vi "Autopatch-v2.3_focus.vi"() -> ()   [LabVIEW 2018]
uses:
  <vilib>/userdefined/High Color/IMAQdx.ctl
  <vilib>/DAQmx/write.llb/DAQmx Write (Analog DBL 1Chan 1Samp).vi
  <vilib>/DAQmx/write.llb/DAQmx Write (Analog Wfm 1Chan NSamp).vi
  <vilib>/DAQmx/read.llb/DAQmx Read (Analog Wfm 1Chan NSamp).vi
  <vilib>/Analysis/baseanly.llb/Mean (DBL).vi
  <vilib>/DAQmx/create/channels.llb/DAQmx Create Channel (AO-Voltage-Basic).vi
  <vilib>/DAQmx/miscellaneous.llb/DAQmx Fill In Error Info.vi
  <vilib>/DAQmx/create/channels.llb/DAQmx Create Channel (AI-Voltage-Basic).vi
  <vilib>/DAQmx/configure/timing.llb/DAQmx Timing (Sample Clock).vi
  <vilib>/DAQmx/configure/trigger.llb/DAQmx Start Trigger (Digital Edge).vi
  <vilib>/Waveform/WDTOps.llb/WDT Waveform Duration DBL.vi
  <vilib>/addons/control/pid/pid.llb/PID (DBL).vi
  <vilib>/vision/driver/NI_Vision_Acquisition_Software.lvlib
  <resource>/objmgr/daqmx.rc
  <vilib>/Analysis/NI_AALBase.lvlib
  <vilib>/measure/NI_MABase.lvlib
  <vilib>/vision/NI_Vision_Development_Module.lvlib
  <vilib>/addons/control/pid/NI_PID_pid.lvlib
  <vilib>/Analysis/NI_AALPro.lvlib
panel:
  out "裁剪数组":i32[](array[numeric])
  in  "模板分数":sgl=650.0
  out "自动接触状态":i32
  in  "没有细胞":bool=TRUE
  out "x+y":sgl
  in  "z输入":dbl=24364.6
  in  "y输入":dbl=3592.0
  in  "x输入":dbl=-28569.0
  in  "二值化":bool=TRUE
  in  "背景图":path=path "D:/韩宇/程序/自动膜片钳系统/img.png"
  in  "Number of Erosion":i32=10
  out "已发送图像":bool
  out "上升找针次数":i32
  in  "升Z轴找针状态机":u16(ring) items=["升Z轴找针初始", "升Z轴找针循环", "升Z轴找针结束"]
  out "物镜下降次数":i32
  in  "发送次数":dbl
  in  "目标细胞位置":bool=TRUE
  out "错误输出 2":errorcluster caption="错误输出"
  out "已强制转换(y)":dbl
  out "已强制转换(x)":dbl
  out "调焦值上升过？":bool
  out "right_old":dbl
  out "Matches 2":T1(array[cluster]) {"Bounding Box"."y" format="%.2f"; "Bounding Box"."x" format="%.2f"; "Position"."y" format="%.2f"; "Position"."x" format="%.2f"; "Score" format="%.2f"; "Scale" format="%.2f"; "Angle" format="%.2f"}
  in  "基路径40":path=path "D:/韩宇/程序/CCD/模板40倍.jpg"
  out "Particle Measurements (Pixels) 2":dbl[][](array[numeric]) format="%.2f"
  in  "Pixel Measurements 2":T2[](array[typedef])=[2] items=["Center of Mass X", "Center of Mass Y", "First Pixel X", "First Pixel Y", "Bounding Rect Left", "Bounding Rect Top", "Bounding Rect Right", "Bounding Rect Bottom", "Max Feret Diameter Start X", "Max Feret Diameter Start Y", "Max Feret Diameter End X", "Max Feret Diameter End Y", "Max Horiz. Segment Length Left", "Max Horiz. Segment Length Right", "Max Horiz. Segment Length Row", "-", "Bounding Rect Width", "Bounding Rect Height", "Bounding Rect Diagonal", "Perimeter", "Convex Hull Perimeter", "Holes' Perimeter", "Max Feret Diameter", "Equivalent Ellipse Major Axis", "Equivalent Ellipse Minor Axis", "Equivalent Ellipse Minor Axis (Feret)", "Equivalent Rect Long Side", "Equivalent Rect Short Side", "Equivalent Rect Diagonal", "Equivalent Rect Short Side (Feret)", "Average Horiz. Segment Length", "Average Vert. Segment Length", "Hydraulic Radius", "Waddel Disk Diameter", "-", "Area", "Holes' Area", "Particle & Holes' Area", "Convex Hull Area", "Image Area", "-", "Number of Holes", "Number of Horiz. Segments", "Number of Vert. Segments", "-", "Orientation", "Max Feret Diameter Orientation", "-", "% Area/Image Area", "% Area/(Particle & Holes' Area)", "Ratio of Equivalent Ellipse Axes", "Ratio of Equivalent Rect Sides", "-", "Elongation Factor", "Compactness Factor", "Heywood Circularity Factor", "Type Factor", "-", "Sum X", "Sum Y", "Sum XX", "Sum XY", "Sum YY", "Sum XXX", "Sum XXY", "Sum XYY", "Sum YYY", "-", "Moment of Inertia XX", "Moment of Inertia XY", "Moment of Inertia YY", "Moment of Inertia XXX", "Moment of Inertia XXY", "Moment of Inertia XYY", "Moment of Inertia YYY", "Norm. Moment of Inertia XX", "Norm. Moment of Inertia XY", "Norm. Moment of Inertia YY", "Norm. Moment of Inertia XXX", "Norm. Moment of Inertia XXY", "Norm. Moment of Inertia XYY", "Norm. Moment of Inertia YYY", "Hu Moment 1", "Hu Moment 2", "Hu Moment 3", "Hu Moment 4", "Hu Moment 5", "Hu Moment 6", "Hu Moment 7"]
  out "傅里叶最大值":dbl
  out "傅里叶数组":bool[](array[boolean])
  in  "傅里叶状态机":u16(ring) items=["傅里叶初始", "傅里叶循环", "傅里叶暂停", "傅里叶结束"]
  out "图像检测到":bool=TRUE
  out "自动封接开始时间":u32
  out "针下降次数":i32
  in  "自动测试":bool
  in  "图像检测":bool
  out "写入的字节":i32
  out "数据输出 3":string
  out "X 3":i32
  out "Y 3":i32
  out "error IO":errorcluster
  out "Y 2":i32
  out "X 2":i32
  in  "针尖移动 2":bool
  in  "升Z轴找针":bool
  in  "傅里叶":bool
  in  "自动对焦状态机":u16(ring) items=["自动对焦初始", "自动对焦循环", "自动对焦结束"]
  in  "自动扫描状态机":u16(ring) items=["自动扫描初始", "自动扫描循环", "自动扫描结束"]
  out "startY":dbl
  in  "手动暂停":bool
  out "Particle Measurements (Pixels)":dbl[][](array[numeric]) format="%.2f"
  in  "Pixel Measurements":T2[](array[typedef])=[3] items=["Center of Mass X", "Center of Mass Y", "First Pixel X", "First Pixel Y", "Bounding Rect Left", "Bounding Rect Top", "Bounding Rect Right", "Bounding Rect Bottom", "Max Feret Diameter Start X", "Max Feret Diameter Start Y", "Max Feret Diameter End X", "Max Feret Diameter End Y", "Max Horiz. Segment Length Left", "Max Horiz. Segment Length Right", "Max Horiz. Segment Length Row", "-", "Bounding Rect Width", "Bounding Rect Height", "Bounding Rect Diagonal", "Perimeter", "Convex Hull Perimeter", "Holes' Perimeter", "Max Feret Diameter", "Equivalent Ellipse Major Axis", "Equivalent Ellipse Minor Axis", "Equivalent Ellipse Minor Axis (Feret)", "Equivalent Rect Long Side", "Equivalent Rect Short Side", "Equivalent Rect Diagonal", "Equivalent Rect Short Side (Feret)", "Average Horiz. Segment Length", "Average Vert. Segment Length", "Hydraulic Radius", "Waddel Disk Diameter", "-", "Area", "Holes' Area", "Particle & Holes' Area", "Convex Hull Area", "Image Area", "-", "Number of Holes", "Number of Horiz. Segments", "Number of Vert. Segments", "-", "Orientation", "Max Feret Diameter Orientation", "-", "% Area/Image Area", "% Area/(Particle & Holes' Area)", "Ratio of Equivalent Ellipse Axes", "Ratio of Equivalent Rect Sides", "-", "Elongation Factor", "Compactness Factor", "Heywood Circularity Factor", "Type Factor", "-", "Sum X", "Sum Y", "Sum XX", "Sum XY", "Sum YY", "Sum XXX", "Sum XXY", "Sum XYY", "Sum YYY", "-", "Moment of Inertia XX", "Moment of Inertia XY", "Moment of Inertia YY", "Moment of Inertia XXX", "Moment of Inertia XXY", "Moment of Inertia XYY", "Moment of Inertia YYY", "Norm. Moment of Inertia XX", "Norm. Moment of Inertia XY", "Norm. Moment of Inertia YY", "Norm. Moment of Inertia XXX", "Norm. Moment of Inertia XXY", "Norm. Moment of Inertia XYY", "Norm. Moment of Inertia YYY", "Hu Moment 1", "Hu Moment 2", "Hu Moment 3", "Hu Moment 4", "Hu Moment 5", "Hu Moment 6", "Hu Moment 7"]
  in  "手动换物镜":bool
  out "扫描变量":dbl=10.0
  in  "自动扫描":bool
  in  "移至工作位置":bool
  out "Z":dbl
  out "Y":dbl
  out "X":dbl
  out "自动接触初始":i32
  in  "枚举":enum16{"200ms", "500ms", "1000ms", ""}(ring)=enum."1000ms"
  out "dX/dt":dbl[](array[numeric])
  in  "下降/向右":bool
  in  "down":bool
  in  "up":bool
  out "Z轴坐标":string
  in  "调焦步伐/um":i64(ring)=3 items=["1", "10", "100", "1000", "10000"]
  in  "停止运动":bool
  in  "设置移动步长":bool
  in  "返回Z轴坐标":bool
  out "x*y":dbl
  out "电阻值":dbl
  in  "钳制电位":i16(ring) items=["0mv", "-70mv"]
  out "起始破膜时间":u32
  in  "自动破膜":bool
  in  "控制箱刺激ON\n/放大器刺激":bool=TRUE
  in  "自动封接":bool
  in  "保存数据":bool
  out "没匹配到？":bool
  in  "PID gains":T3={"proportional gain (Kc)"=-0.05, "integral time (Ti, min)"=0.0, "derivative time (Td, min)"=0.0} caption="PID增益" {"derivative time (Td, min)" format="%.3f"; "integral time (Ti, min)" format="%.3f"; "proportional gain (Kc)" format="%.3f"}
  in  "PID gains 2":T3={"proportional gain (Kc)"=0.05, "integral time (Ti, min)"=0.0, "derivative time (Td, min)"=0.0} caption="PID增益" {"derivative time (Td, min)" format="%.3f"; "integral time (Ti, min)" format="%.3f"; "proportional gain (Kc)" format="%.3f"}
  out "对焦变量":dbl
  in  "下降步伐/um":dbl=1.0
  in  "自动接触":bool
  out "傅里叶求和":sgl(graph)
  in  "针尖移动":bool
  in  "针尖细对焦":bool
  in  "针尖粗对焦":bool
  out "二值化":T4(plugin-control)
  in  "Range":cluster{"Lower value":sgl, "Upper value":sgl}={"Lower value"=10.0, "Upper value"=255.0} {"Upper value" format="%.2f"; "Lower value" format="%.2f"}
  in  "Operation":T5(ring)=enum."Dilate"
  out "Right":dbl
  out "目标坐标":i32[](array[numeric])
  in  "针尖模板匹配":bool=TRUE
  in  "基路径20":path=path "D:/韩宇/程序/CCD/针尖水下模板20X.jpg"
  out "Number of Matches":i32
  in  "Minimum Contrast":i32 min=0 max=255 step=1
  in  "Minimum Match Score":sgl=600.0 min=0 max=1000 format="%.2f"
  in  "Number of Matches Requested":i32=1 min=1
  in  "Match Mode":u16(ring) items=["Shift Invariant", "Rotation Invariant"]
  out "针尖坐标":sgl[](array[numeric])
  in  "入液阻值校准":bool
  out "校准的入液阻值":dbl
  out "错误输出 3":errorcluster caption="错误输出"
  in  "低负开关":bool
  in  "低正开关":bool
  in  "大气压":bool
  in  "高负开关":bool
  in  "高正开关":bool
  in  "case":dbl
  out "测量值":dbl
  out "给定值":dbl
  out "输出气压波形图表":cluster{dbl, "低负":dbl}(graph)
  in  "低负":sgl(knob)=-0.45548448
  in  "高负":sgl(knob)=-5.0
  in  "低正":sgl(knob)=0.49642125 scale=0.0..2.0
  in  "高正":sgl(knob)=10.718505 scale=0.0..15.0
  in  "采样率":u32=255
  in  "DevIndex":i32
  in  "Holding Voltage":dbl=-70.0
  out "Negative Peak":dbl
  out "阻值波形图表":dbl(graph)
  out "Resistance(MΩ)":dbl
  out "！":bool
  in  "电压钳/电流钳":u16(ring) items=["Voltage Clamp", "Current Clamp"]
  out "电流信号波形图":waveform(dbl)(graph)
  in  "frequency":dbl=20.0
  in  "Averaging":i32=5
  in  "amplitude":dbl=0.01
  in  "阻值数组":dbl[](array[numeric])
  out "循环时间":u32
  out "Image":T4(plugin-control)
  out "错误输出":errorcluster
  in  "停止":bool
  in  "Session In":T6="cam1"
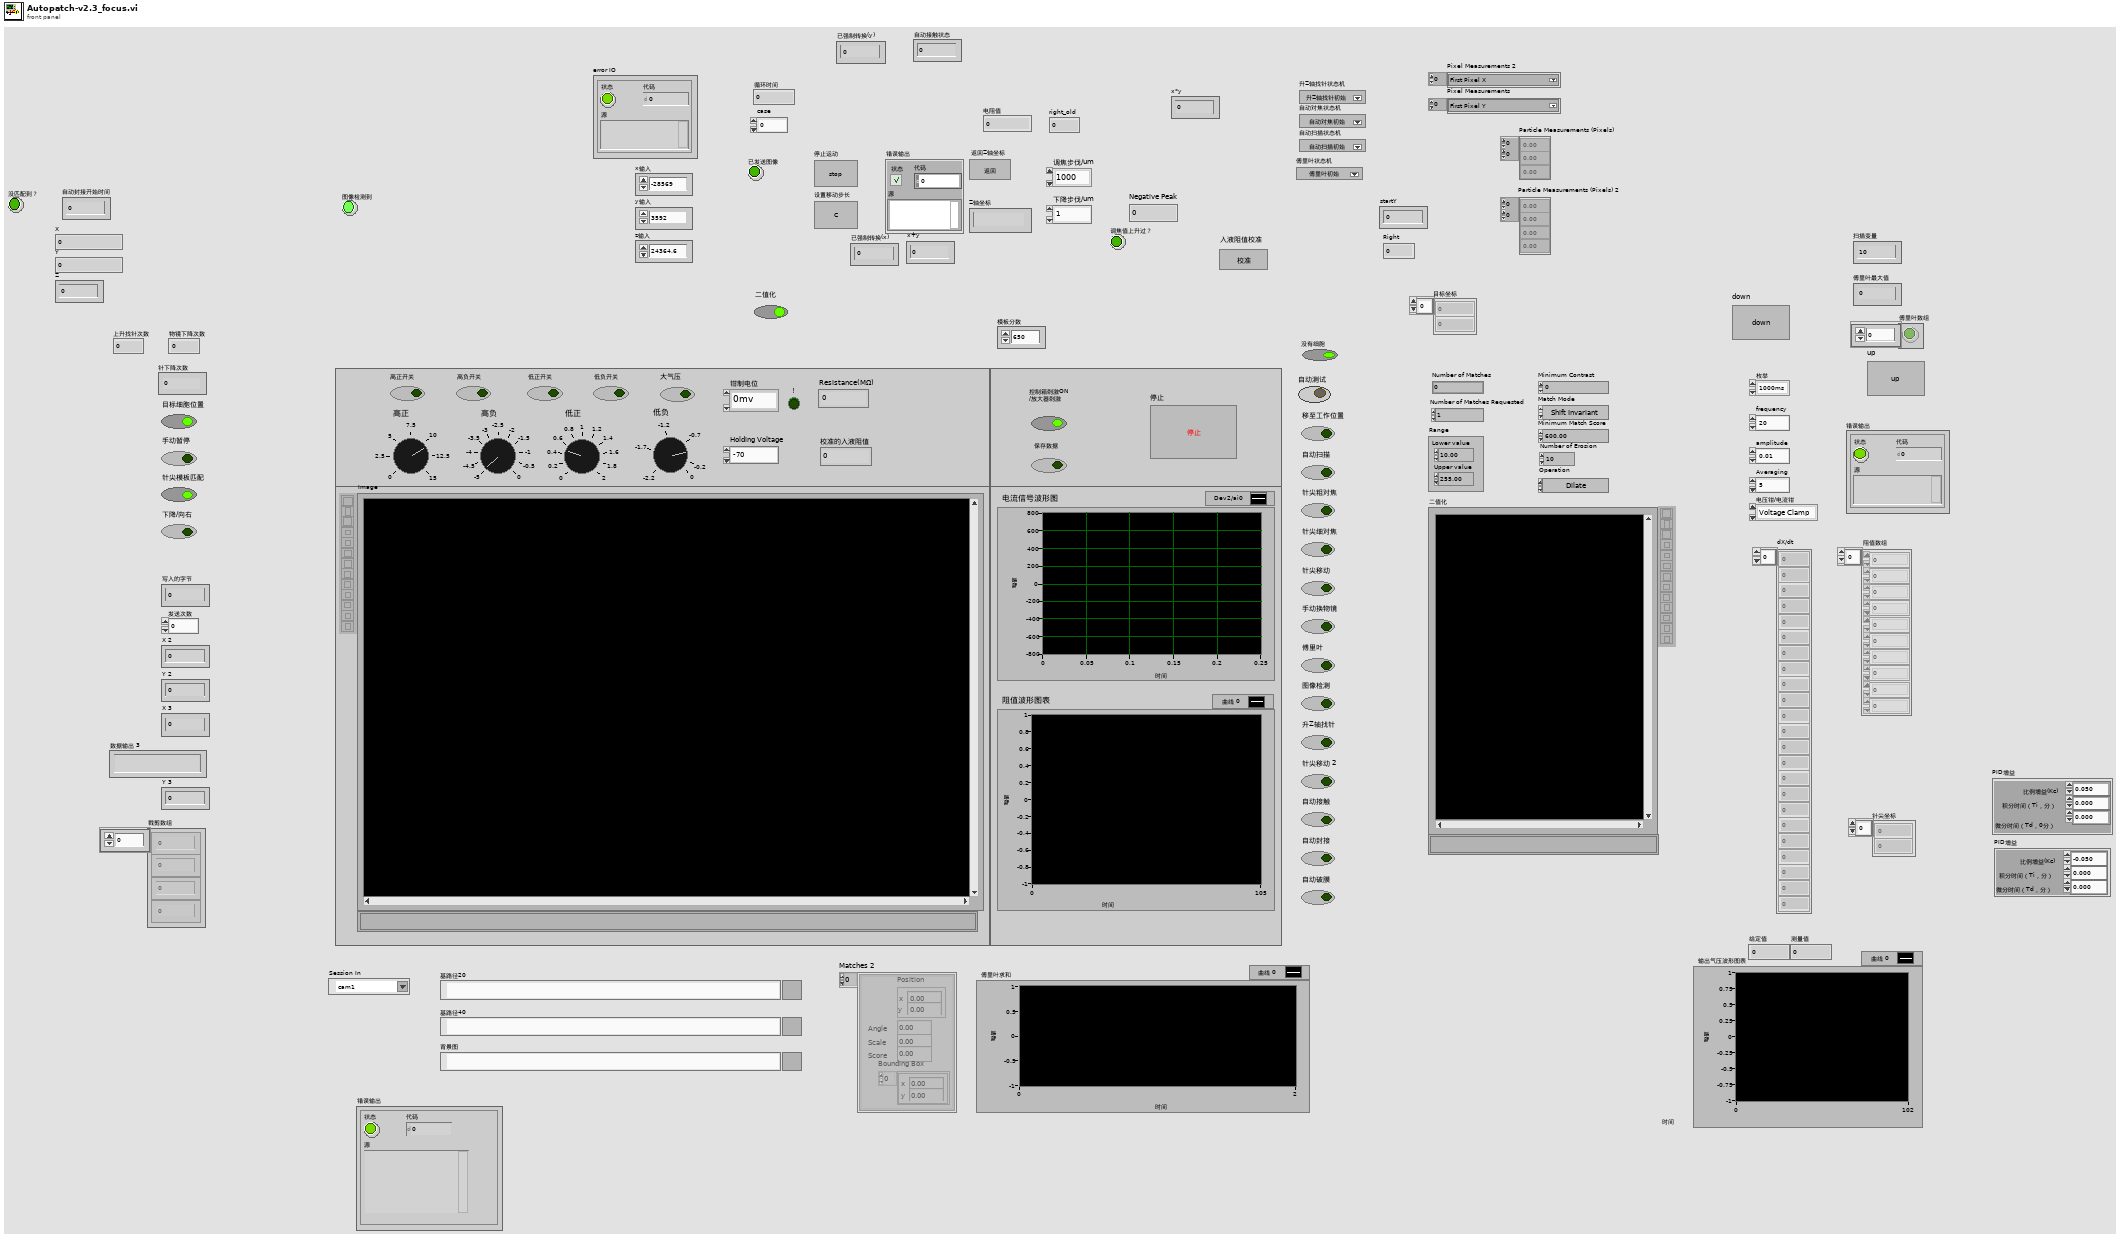
[diagram p1: front panel]
types:
  T1 = cluster{"Position":cluster{"x":sgl, "y":sgl}, "Angle":sgl, "Scale":sgl, "Score":sgl, "Bounding Box":cluster{"x":sgl, "y":sgl}[]}[]
  T2 = typedef "Particle Parameters" = i32
  T3 = cluster{"proportional gain (Kc)":dbl, "integral time (Ti, min)":dbl, "derivative time (Td, min)":dbl}
  T4 = typedef "IMAQ Image.ctl" = refnum<image>
  T5 = enum32{"AutoM", "Close", "Dilate", "Erode", "Gradient", "Gradient out", "Gradient in", "Hit miss", "Open", "PClose", "POpen", "Thick", "Thin"}
  T6 = typedef "IMAQdx.ctl" = refnum<k21>
  T7 = typedef "Image Type" = u32
  T8 = enum16{"open", "replace", "create", "open or create", "replace or create", "replace or create with confirmation"}
  T9 = cluster{"Averaging":i32, "frequency":dbl, "amplitude":dbl, "Proportion":dbl, "Fs":dbl}
  T10 = enum16{"Sine Wave", "Triangle Wave", "Square Wave", "Sawtooth Wave"}
  T11 = cluster{"Position":cluster{"x":sgl, "y":sgl}, "Angle":sgl, "Scale":sgl, "Score":sgl, "Bounding Box":cluster{"x":sgl, "y":sgl}[]}
  T12 = enum32{"Real", "Imaginary", "Magnitude", "Phase"}
  T13 = cluster{"Global Rectangle":i32[], "Contours":cluster{"Contour Type":u32, "ROI Type":u32, "Points":i32[]}[]}
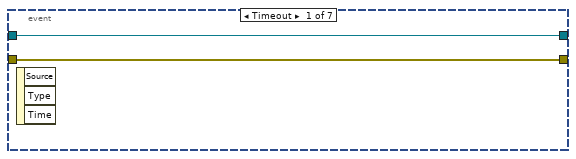
[diagram p3: hidden frame]
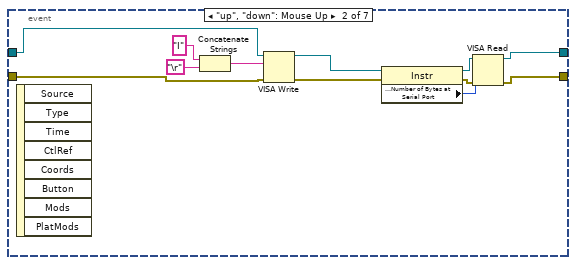
[diagram p4: hidden frame]
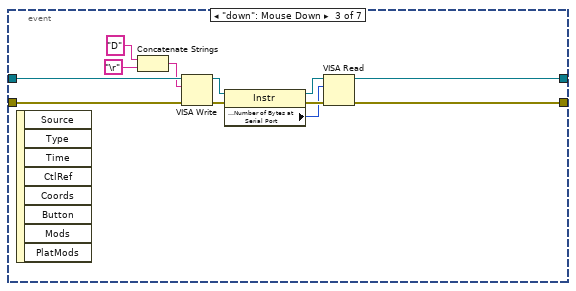
[diagram p5: hidden frame]
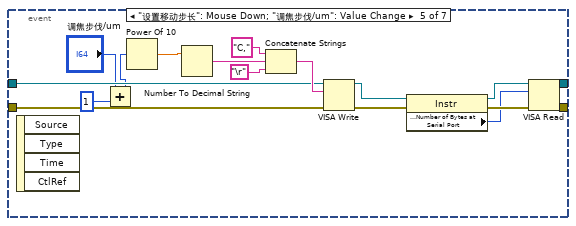
[diagram p6: hidden frame]
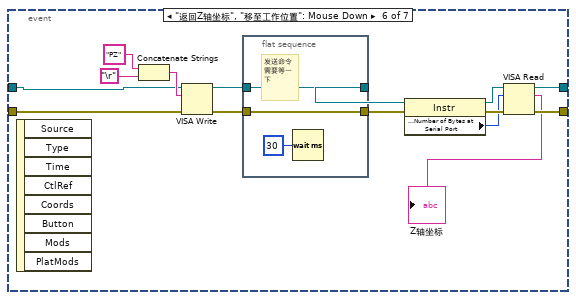
[diagram p7: hidden frame]
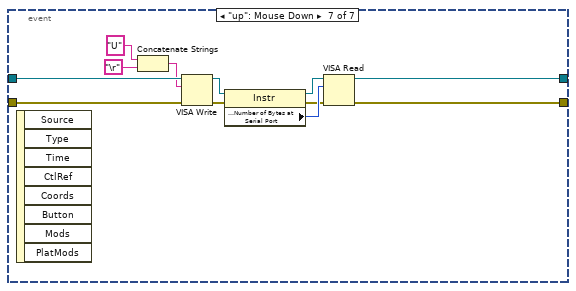
[diagram p8: hidden frame]
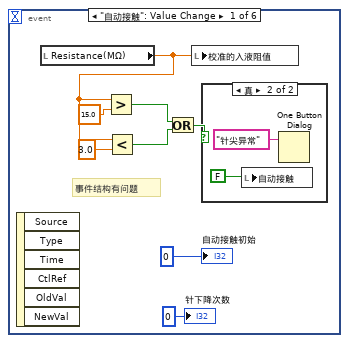
[diagram p11: hidden frame]
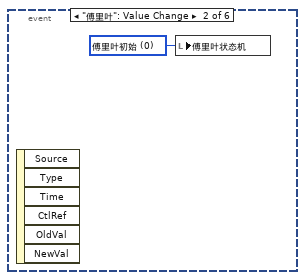
[diagram p13: hidden frame]
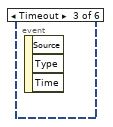
[diagram p14: hidden frame]
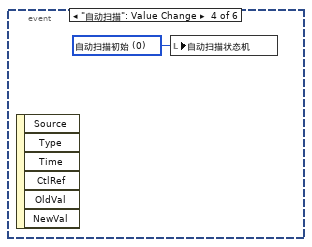
[diagram p15: hidden frame]
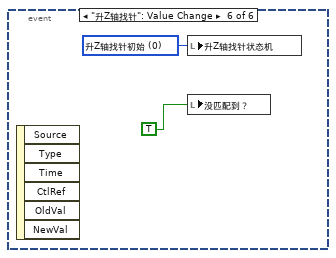
[diagram p16: hidden frame]
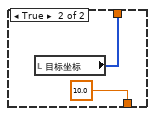
[diagram p17: hidden frame]
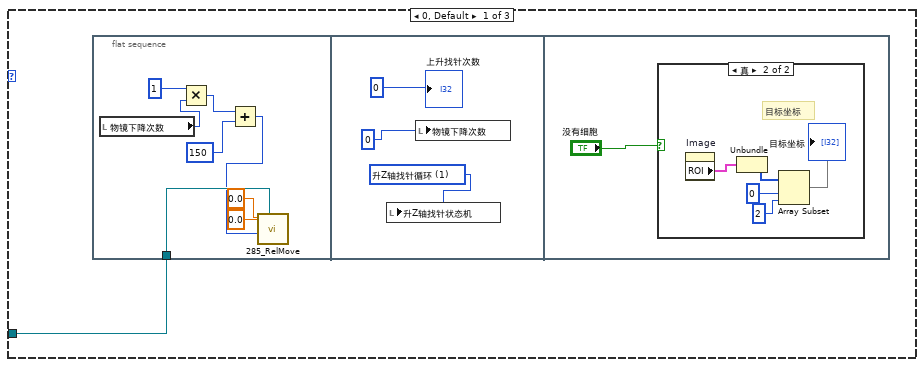
[diagram p19: hidden frame]
diagram:
  w4 = T7 0 items=["Grayscale (U8)", "Grayscale (I16)", "Grayscale (SGL)", "Complex (CSG)", "RGB (U32)", "HSL (U32)", "RGB (U64)", "Grayscale (U16)"] ("Image Type")
  w11 = T7 0 items=["Grayscale (U8)", "Grayscale (I16)", "Grayscale (SGL)", "Complex (CSG)", "RGB (U32)", "HSL (U32)", "RGB (U64)", "Grayscale (U16)"] ("Image Type")
  w19 = T7 0 items=["Grayscale (U8)", "Grayscale (I16)", "Grayscale (SGL)", "Complex (CSG)", "RGB (U32)", "HSL (U32)", "RGB (U64)", "Grayscale (U16)"] ("Image Type")
  w30 = T7 3 items=["Grayscale (U8)", "Grayscale (I16)", "Grayscale (SGL)", "Complex (CSG)", "RGB (U32)", "HSL (U32)", "RGB (U64)", "Grayscale (U16)"] ("Image Type")
  w28 = T7 3 items=["Grayscale (U8)", "Grayscale (I16)", "Grayscale (SGL)", "Complex (CSG)", "RGB (U32)", "HSL (U32)", "RGB (U64)", "Grayscale (U16)"] ("Image Type")
  w82 = T7 0 items=["Grayscale (U8)", "Grayscale (I16)", "Grayscale (SGL)", "Complex (CSG)", "RGB (U32)", "HSL (U32)", "RGB (U64)", "Grayscale (U16)"] ("Image Type")
  w96 = FALSE
  # "XY移动平台"
  # "Mp285"
  # "保存数据"
  n1 = case shown="真" "自动测试" {
    frame False {
    }
    frame True {
      n2 = flat-sequence {
        frame #0 {
          # "每换一次针，\n，请连接网，需要标定初始位置，\n并保存针尖20倍水下模板\n和40倍水下模板，\n以及背景图,调节二值化阈值\n并将针尖移动细胞表面上方,"
          n3 = One Button Dialog(message="请安装玻璃电极并手动更换20倍显微镜" ("消息")) -> ()  [unwired: 1 in, 1 out]
        }
        frame #1 {
          w158 = TRUE ("自动移至工作位置")
          n4 = local write "针尖粗对焦"(FALSE ("针尖粗对焦")) -> ()
          n5 = local write "针尖细对焦"(FALSE ("针尖细对焦")) -> ()
          n6 = local write "傅里叶"(FALSE ("傅里叶")) -> ()
          n7 = local write "移至工作位置"(w158) -> ()
          n8 = local write "针尖移动"(FALSE ("针尖自动移动")) -> ()
          n9 = local write "低正开关"(w158) -> ()
          n10 = local write "针尖移动 2"(FALSE ("针尖自动移动 2")) -> ()
          n11 = local write "自动扫描"(FALSE ("自动扫描")) -> ()
          n12 = local write "手动换物镜"(FALSE ("手动换物镜")) -> ()
          n13 = local write "自动接触"(FALSE ("自动接触")) -> ()
          n14 = local write "升Z轴找针"(FALSE ("升Z轴找针")) -> ()
          n15 = local write "目标坐标"(i32[] [0, 0] ("目标坐标")) -> ()
        }
      }
    }
  }
  n16 = flat-sequence {
    tunnel: [w171] -> w143
    frame #0 {
      # "选择刺激方式，内部刺激更准"
      n17 = Array Size(array="阻值数组") -> (size(s)=w170:i32)
      n18 = Delete From Array(array="阻值数组", length=w170) -> (array with subset deleted=w168:dbl[])  [unwired: 1 in, 1 out]
      n19 = local write "阻值数组"(w168) -> ()
    }
    frame #1 {
      # "波形个数"
      # "计算电阻波形比例"
      n20 = Bundle("Averaging"="Averaging", "frequency"="frequency", "amplitude"="amplitude", "Proportion"=0.4, "Fs"=20000.0) -> (w171:T9)  [unwired: 1 in]
    }
  }
  n21 = call "OpenDevice.vi"("DevIndex"="DevIndex") -> ("错误输出"=w123:errorcluster, "DevIndex Output"=w121:i32)  [unwired: 9 in]
  n22 = call "SetUSB2AiRange.vi"("错误输入（无错误）"=w123, "Range"=sgl 5.0, "DevIndex"=w121) -> ("错误输出"=w132:errorcluster, "DevIndex Output"=w130:i32)  [unwired: 7 in]
  n23 = call <vilib>:"IMAQdx Open Camera.vi"("Session In"="Session In") -> ("error out"=w155:errorcluster, "Session Out"=w152:T6)  [unwired: 9 in]
  n24 = call "IMAQ Create"("Image Name"="", "Image Type"=w4) -> ("New Image"=w5:T4)  [unwired: 3 in, 1 out]
  n25 = call "IMAQ Create"("Image Name"="针尖模板40倍", "Image Type"=w19) -> ("New Image"=w18:T4)  [unwired: 3 in, 1 out]
  n26 = Obtain Queue(element data type=FALSE) -> (queue out=w41:refnum<queue>, error out=w40:errorcluster)  [unwired: 4 in, 1 out]
  n27 = call "IMAQ Create"("Image Name"="针尖模板20倍", "Image Type"=w82) -> ("New Image"=w83:T4)  [unwired: 3 in, 1 out]
  n28 = call "SetSampleRate.vi"("错误输入（无错误）"=w132, "SampleRate"="采样率", "DevIndex"=w130) -> ("错误输出"=w133:errorcluster, "DevIndex Output"=w131:i32)  [unwired: 7 in]
  n29 = call "IMAQ ReadFile 2"("File Path"="背景图", "Image"=w5) -> ("Image Out"=w3:T4)  [unwired: 5 in, 4 out]
  n30 = call "IMAQ ReadFile 2"("File Path"="基路径40", "Image"=w18) -> ("Image Out"=w16:T4)  [unwired: 5 in, 4 out]
  n31 = call "IMAQ ReadFile 2"("File Path"="基路径20", "Image"=w83) -> ("Image Out"=w81:T4)  [unwired: 5 in, 4 out]
  n32 = call <vilib>:"IMAQdx Configure Grab.vi"("error in"=w155, "Session In"=w152) -> ("error out"=w140:errorcluster, "Session Out"=w153:T6)  [unwired: 8 in]
  n33 = call "SetTrigSource.vi"("错误输入（无错误）"=w133, "TrigSource"=u8 0, "DevIndex"=w131) -> ("错误输出"=w128:errorcluster, "DevIndex Output"=w127:i32)  [unwired: 7 in]
  n34 = call "IMAQ Create"("Image Name"="原图像") -> ("New Image"=w151:T4, "error out"=w138:errorcluster)  [unwired: 4 in]
  n35 = call "IMAQ Create"("Image Name"="灰度图") -> ("New Image"=w144:T4)  [unwired: 4 in, 1 out]
  n36 = call "SetSoftTrig.vi"("错误输入（无错误）"=w128, "Trig"=u8 1, "DevIndex"=w127) -> ("错误输出"=w124:errorcluster, "DevIndex Output"=w122:i32)  [unwired: 7 in]
  n37 = call "285_Initialize.vi"() -> ("VISA资源名称输出"=w39:refnum<visa-resource-name>)  [unwired: 10 in, 1 out]
  n38 = call "285_Initialize_1.vi"() -> ("VISA资源名称输出"=w38:refnum<visa-resource-name>)  [unwired: 10 in, 1 out]
  n39 = call "InitDA.vi"("错误输入（无错误）"=w124, "DevIndex"=w122) -> ("错误输出"=w118:errorcluster, "DevIndex Output"=w119:i32)  [unwired: 8 in]
  n40 = call "PRIOR_Initialize.vi"() -> ("错误输出"=w37:errorcluster, "VISA资源名称输出"=w33:refnum<visa-resource-name>)  [unwired: 10 in]
  n41 = while {
    tunnel: w33 -> [w186]
    tunnel: [w183] -> w42
    tunnel: [w187] -> w43
    tunnel: w41 -> [w180]
    tunnel: w40 -> [w179]
    tunnel: w37 -> [w177]
    stop <- w178 stop-if-true
    n42 = VISA Flush I/O Buffer(VISA resource name=w186, error in (no error)=w177) -> (VISA resource name out=w185:refnum<visa-resource-name>, error out=w184:errorcluster)  [unwired: 1 in]
    n43 = Dequeue Element(queue=w180, timeout in ms (-1)=1 ("超时毫秒(-1)"), error in (no error)=w179) -> (error out=w182:errorcluster)  [unwired: 3 out]
    n44 = event shown="[3] \"停止运动\": 鼠标按下" {
      selector: _ -> [_ _ _ _ _ _ _]
      dyn-events: _ -> [_ _ _ _ _ _ _]
      timeout: 1 -> [_ _ _ _ _ _ _]
      tunnel: [w190 w192 w214 w216 w234 w250 w273] -> w187
      tunnel: [w189 w191 w213 w215 w233 w249 w272] -> w183
      tunnel: w185 -> [w190 w194 w212 w218 w236 w252 w271]
      tunnel: w184 -> [w189 w193 w211 w217 w235 w251 w270]
      event Timeout {
        n45 = event-data() -> ()  [unwired: 1 in, 3 out]
      }
      event "up", "down": Mouse Up {
        n46 = event-data() -> ()  [unwired: 1 in, 8 out]
        n47 = Concatenate Strings("I" ("写入缓冲区"), "\r") -> (w202:string)
        n48 = VISA Write ("VISA写入")(VISA resource name=w194, write buffer=w202, error in (no error)=w193) -> (VISA resource name out=w196:refnum<visa-resource-name>, error out=w195:errorcluster)  [unwired: 1 out]
        n49 = property class="Instr"(reference=w196, error in=w195) -> (reference out=w197:refnum<visa-resource-name>, error out=w198:errorcluster, "Serial Settings:Number of Bytes at Serial Port"=w199:u32)
        n50 = VISA Read(VISA resource name=w197, byte count=w199, error in (no error)=w198) -> (VISA resource name out=w192:refnum<visa-resource-name>, error out=w191:errorcluster)  [unwired: 2 out]
      }
      event "down": Mouse Down {
        n51 = event-data() -> ()  [unwired: 1 in, 8 out]
        n52 = Concatenate Strings("D" ("写入缓冲区"), "\r") -> (w203:string)
        n53 = VISA Write ("VISA写入")(VISA resource name=w212, write buffer=w203, error in (no error)=w211) -> (VISA resource name out=w209:refnum<visa-resource-name>, error out=w210:errorcluster)  [unwired: 1 out]
        n54 = property class="Instr"(reference=w209, error in=w210) -> (reference out=w208:refnum<visa-resource-name>, error out=w207:errorcluster, "Serial Settings:Number of Bytes at Serial Port"=w206:u32)
        n55 = VISA Read(VISA resource name=w208, byte count=w206, error in (no error)=w207) -> (VISA resource name out=w214:refnum<visa-resource-name>, error out=w213:errorcluster)  [unwired: 2 out]
      }
      event "停止运动": Mouse Down {
        n56 = event-data() -> ()  [unwired: 1 in, 8 out]
        n57 = Concatenate Strings("I" ("写入缓冲区"), "\r") -> (w219:string)
        n58 = VISA Write ("VISA写入")(VISA resource name=w218, write buffer=w219, error in (no error)=w217) -> (VISA resource name out=w225:refnum<visa-resource-name>, error out=w226:errorcluster)  [unwired: 1 out]
        n59 = property class="Instr"(reference=w225, error in=w226) -> (reference out=w224:refnum<visa-resource-name>, error out=w223:errorcluster, "Serial Settings:Number of Bytes at Serial Port"=w222:u32)
        n60 = VISA Read(VISA resource name=w224, byte count=w222, error in (no error)=w223) -> (VISA resource name out=w216:refnum<visa-resource-name>, error out=w215:errorcluster)  [unwired: 2 out]
      }
      event "设置移动步长": Mouse Down; "调焦步伐/um": Value Change {
        n61 = event-data() -> ()  [unwired: 1 in, 4 out]
        n62 = Add(x="调焦步伐/um", y=i64 1) -> (x+y=w227:i64)
        n63 = Power Of 10(x=w227) -> (10^x=w230:dbl)
        n64 = Number To Decimal String(number=w230) -> (decimal integer string=w231:string)  [unwired: 1 in]
        n65 = Concatenate Strings("C," ("写入缓冲区"), w231, "\r") -> (w237:string)
        n66 = VISA Write ("VISA写入")(VISA resource name=w236, write buffer=w237, error in (no error)=w235) -> (VISA resource name out=w242:refnum<visa-resource-name>, error out=w243:errorcluster)  [unwired: 1 out]
        n67 = property class="Instr"(reference=w242, error in=w243) -> (reference out=w241:refnum<visa-resource-name>, error out=w240:errorcluster, "Serial Settings:Number of Bytes at Serial Port"=w239:u32)
        n68 = VISA Read(VISA resource name=w241, byte count=w239, error in (no error)=w240) -> (VISA resource name out=w234:refnum<visa-resource-name>, error out=w233:errorcluster)  [unwired: 2 out]
      }
      event "返回Z轴坐标", "移至工作位置": Mouse Down {
        n69 = event-data() -> ()  [unwired: 1 in, 8 out]
        n70 = Concatenate Strings("PZ" ("写入缓冲区"), "\r") -> (w254:string)
        n71 = VISA Write ("VISA写入")(VISA resource name=w252, write buffer=w254, error in (no error)=w251) -> (VISA resource name out=w248:refnum<visa-resource-name>, error out=w247:errorcluster)  [unwired: 1 out]
        n72 = flat-sequence {
          tunnel: w248 -> [w260]
          tunnel: w247 -> [w261]
          tunnel: [w261] -> w245
          tunnel: [w260] -> w246
          frame #0 {
            # "发送命令需要等一下"
            n73 = Wait (ms)(milliseconds to wait=u32 30 ("等待时间（毫秒）")) -> ()  [unwired: 1 out]
          }
        }
        n74 = property class="Instr"(reference=w246, error in=w245) -> (reference out=w258:refnum<visa-resource-name>, error out=w257:errorcluster, "Serial Settings:Number of Bytes at Serial Port"=w256:u32)
        n75 = VISA Read(VISA resource name=w258, byte count=w256, error in (no error)=w257) -> (VISA resource name out=w250:refnum<visa-resource-name>, read buffer=→"Z轴坐标":string, error out=w249:errorcluster)  [unwired: 1 out]
      }
      event "up": Mouse Down {
        n76 = event-data() -> ()  [unwired: 1 in, 8 out]
        n77 = Concatenate Strings("U" ("写入缓冲区"), "\r") -> (w267:string)
        n78 = VISA Write ("VISA写入")(VISA resource name=w271, write buffer=w267, error in (no error)=w270) -> (VISA resource name out=w266:refnum<visa-resource-name>, error out=w265:errorcluster)  [unwired: 1 out]
        n79 = property class="Instr"(reference=w266, error in=w265) -> (reference out=w263:refnum<visa-resource-name>, error out=w262:errorcluster, "Serial Settings:Number of Bytes at Serial Port"=w264:u32)
        n80 = VISA Read(VISA resource name=w263, byte count=w264, error in (no error)=w262) -> (VISA resource name out=w273:refnum<visa-resource-name>, error out=w272:errorcluster)  [unwired: 2 out]
      }
    }
    n81 = Unbundle By Name(w182) -> ("status"=w178:bool)
  }
  n82 = while {
    tunnel: w119 -> [w286]
    tunnel: w41 -> [w325]
    tunnel: w40 -> [w324]
    tunnel: [w278] -> w45
    tunnel: w118 -> [w285]
    tunnel: [w276] -> w44
    stop <- w321 stop-if-true
    # "气压控制循环"
    # "气压到电压转换"
    n83 = Dequeue Element(queue=w325, timeout in ms (-1)=1 ("超时毫秒(-1)"), error in (no error)=w324) -> (error out=w322:errorcluster)  [unwired: 3 out]
    n84 = Unbundle By Name(w322) -> ("status"=w321:bool)
    n85 = In Range and Coerce(upper limit=sgl 15.0 ("上限"), x="高正", lower limit=sgl 0.0 ("下限")) -> (coerced(x)=w289:sgl)  [unwired: 1 out]
    n86 = In Range and Coerce(upper limit=sgl 0.0 ("上限"), x="高负", lower limit=sgl -5.0 ("下限")) -> (coerced(x)=w293:sgl)  [unwired: 1 out]
    n87 = Divide(x=w289, y=3) -> (x/y=w310:sgl)
    n88 = Divide(x=w293, y=-1.004) -> (x/y=w306:dbl)
    n89 = In Range and Coerce(upper limit=sgl 2.0 ("上限"), x="低正", lower limit=sgl 0.0 ("下限")) -> (coerced(x)=w297:sgl)  [unwired: 1 out]
    n90 = call "SetDA.vi"("错误输入（无错误）"=w285, "DAVolt"=w310, "DANum"=u8 0, "DevIndex"=w286) -> ("错误输出"=w319:errorcluster, "DevIndex Output"=w320:i32)  [unwired: 6 in]
    n91 = In Range and Coerce(upper limit=sgl 0.0 ("上限"), x="低负", lower limit=sgl -2.2 ("下限")) -> (coerced(x)=w299:sgl)  [unwired: 1 out]
    n92 = call "SetDA.vi"("错误输入（无错误）"=w319, "DAVolt"=w306, "DANum"=u8 1, "DevIndex"=w320) -> ("错误输出"=w318:errorcluster, "DevIndex Output"=w317:i32)  [unwired: 6 in]
    n93 = Multiply(x=w297, y=2.564) -> (x*y=w303:dbl)
    n94 = Multiply(x=w299, y=-2.294) -> (x*y=w304:dbl)
    n95 = call "SetDA.vi"("错误输入（无错误）"=w318, "DAVolt"=w303, "DANum"=u8 2, "DevIndex"=w317) -> ("错误输出"=w315:errorcluster, "DevIndex Output"=w316:i32)  [unwired: 6 in]
    n96 = call "SetDA.vi"("错误输入（无错误）"=w315, "DAVolt"=w304, "DANum"=u8 3, "DevIndex"=w316) -> ("错误输出"=w279:errorcluster, "DevIndex Output"=w280:i32)  [unwired: 6 in]
    n97 = event shown="[2] \"大气压\": 值改变" {
      selector: _ -> [_ _ _ _ _ _ _ _]
      dyn-events: _ -> [_ _ _ _ _ _ _ _]
      timeout: 1 -> [_ _ _ _ _ _ _ _]
      event "高正开关": Value Change {
        n98 = event-data() -> ("OldVal"=w412:bool)  [unwired: 1 in, 5 out]
        n99 = local read "高正开关"() -> (w413:bool)
        n100 = case shown="真" w413 {
          tunnel: w412 -> [_ w415]
          frame False {
          }
          frame True {
            n101 = local write "高负开关"(w415) -> ()
            n102 = local write "低负开关"(w415) -> ()
            n103 = local write "低正开关"(w415) -> ()
            n104 = local write "大气压"(w415) -> ()
            n105 = local write "case"(1.0) -> ()
          }
        }
      }
      event Timeout {
        n106 = event-data() -> ()  [unwired: 1 in, 3 out]
      }
      event "大气压": Value Change {
        n107 = event-data() -> ("OldVal"=w416:bool)  [unwired: 1 in, 5 out]
        n108 = local read "大气压"() -> (w417:bool)
        n109 = case shown="真" w417 {
          tunnel: w416 -> [_ w419]
          frame False {
          }
          frame True {
            n110 = local write "高负开关"(w419) -> ()
            n111 = local write "低正开关"(w419) -> ()
            n112 = local write "低负开关"(w419) -> ()
            n113 = local write "高正开关"(w419) -> ()
            n114 = local write "case"(5.0) -> ()
          }
        }
      }
      event "低正开关": Value Change {
        n115 = event-data() -> ("OldVal"=w421:bool)  [unwired: 1 in, 5 out]
        n116 = local read "低正开关"() -> (w420:bool)
        n117 = case shown="真" w420 {
          tunnel: w421 -> [_ w423]
          frame False {
          }
          frame True {
            n118 = local write "高正开关"(w423) -> ()
            n119 = local write "高负开关"(w423) -> ()
            n120 = local write "低负开关"(w423) -> ()
            n121 = local write "大气压"(w423) -> ()
            n122 = local write "case"(3.0) -> ()
          }
        }
      }
      event "低负开关": Value Change {
        n123 = event-data() -> ("OldVal"=w425:bool)  [unwired: 1 in, 5 out]
        n124 = local read "低负开关"() -> (w424:bool)
        n125 = case shown="真" w424 {
          tunnel: w425 -> [_ w427]
          frame False {
          }
          frame True {
            n126 = local write "高负开关"(w427) -> ()
            n127 = local write "低正开关"(w427) -> ()
            n128 = local write "高正开关"(w427) -> ()
            n129 = local write "大气压"(w427) -> ()
            n130 = local write "case"(4.0) -> ()
          }
        }
      }
      event "高负开关": Value Change {
        n131 = event-data() -> ("OldVal"=w429:bool)  [unwired: 1 in, 5 out]
        n132 = local read "高负开关"() -> (w428:bool)
        n133 = case shown="真" w428 {
          tunnel: w429 -> [_ w431]
          frame False {
          }
          frame True {
            n134 = local write "低正开关"(w431) -> ()
            n135 = local write "低负开关"(w431) -> ()
            n136 = local write "高正开关"(w431) -> ()
            n137 = local write "大气压"(w431) -> ()
            n138 = local write "case"(2.0) -> ()
          }
        }
      }
      event "自动封接": Value Change {
        # "初始值"
        n139 = event-data() -> ()  [unwired: 1 in, 6 out]
        n140 = Tick Count (ms)() -> (millisecond timer value=w432:u32)
        n141 = local write "低负"(-0.66) -> ()
        n142 = local write "自动封接开始时间"(w432) -> ()
      }
      event "自动破膜": Value Change {
        n143 = event-data() -> ()  [unwired: 1 in, 6 out]
        n144 = Tick Count (ms)() -> (millisecond timer value=→"起始破膜时间":u32)
      }
    }
    n145 = case shown="真" "自动封接" {
      frame False {
      }
      frame True {
        w354 = 100.0 ("y")
        w364 = 1300.0 ("y")
        n146 = local read "阻值数组"() -> (w365:dbl[])
        n147 = disable-structure shown="禁用" {
          frame Disabled {
            # "阈值确定？？"
            # "气压微调"
            n148 = local read "阻值数组"() -> (w380:dbl[])
            n149 = call <vilib>:"Derivative x(t).vi"("X"=w380) -> ("dX/dt"=w377:dbl[])  [unwired: 9 in, 1 out]
            "dX/dt" <- w377
            n150 = Index Array(array=w377, index=2 ("索引")) -> (element=w373:dbl)
            n151 = Greater?(x=w373, y=100.0) -> (0:w379:bool)
            n152 = Less?(x=w373, y=10.0) -> (x < y?=w378:bool)
            n153 = case shown="真" w379 {
              frame False {
              }
              frame True {
                n154 = local read "低负"() -> (w388:sgl)
                n155 = Add(x=0.05, y=w388) -> (x+y=w391:dbl)
                n156 = In Range and Coerce(upper limit=0.0, x=w391, lower limit=-1.5) -> (coerced(x)=w387:dbl)  [unwired: 1 out]
                n157 = local write "低负"(w387) -> ()
              }
            }
            n158 = case shown="真" w378 {
              frame False {
              }
              frame True {
                n159 = local read "低负"() -> (w382:sgl)
                n160 = Add(x=-0.05, y=w382) -> (x+y=w385:dbl)
                n161 = In Range and Coerce(upper limit=0.0, x=w385, lower limit=-1.5) -> (coerced(x)=w381:dbl)  [unwired: 1 out]
                n162 = local write "低负"(w381) -> ()
              }
            }
          }
          frame Enabled {
          }
        }
        n163 = Index Array(array=w365, index=0 ("索引")) -> (element=w357:dbl)
        n164 = Index Array(array=w365, index=1 ("索引")) -> (element=w356:dbl)
        n165 = Index Array(array=w365, index=2 ("索引")) -> (element=w355:dbl)
        n166 = Index Array(array=w365, index=3 ("索引")) -> (element=w367:dbl)
        n167 = Index Array(array=w365, index=4 ("索引")) -> (element=w366:dbl)
        n168 = Greater?(x=w357, y=w364) -> (0:w363:bool)
        n169 = Greater?(x=w355, y=w364) -> (0:w361:bool)
        n170 = Greater?(x=w356, y=w364) -> (0:w362:bool)
        n171 = Greater?(x=w367, y=w364) -> (0:w360:bool)
        n172 = Greater?(x=w366, y=w364) -> (0:w359:bool)
        n173 = Compound Arithmetic op=AND ("复合运算")(w363, w362, w361, w360, w359) -> (w358:bool)
        n174 = Greater?(x=w357, y=w354) -> (0:w353:bool)
        n175 = Greater?(x=w356, y=w354) -> (0:w352:bool)
        n176 = Greater?(x=w355, y=w354) -> (0:w351:bool)
        n177 = Compound Arithmetic op=AND ("复合运算")(w353, w352, w351) -> (w350:bool)
        n178 = case shown="真" w350 {
          frame False {
            w393 = i16 0 items=["0mv", "-70mv"] ("钳制电位")
            n179 = local write "钳制电位"(w393) -> ()
          }
          frame True {
            w394 = i16 1 items=["0mv", "-70mv"] ("钳制电位")
            n180 = local write "钳制电位"(w394) -> ()
          }
        }
        n181 = case shown="假" w358 {
          frame True {
            n182 = flat-sequence {
              frame #0 {
                w395 = FALSE
                n183 = local write "高负开关"(w395) -> ()
                n184 = local write "低负开关"(w395) -> ()
                n185 = local write "低正开关"(w395) -> ()
                n186 = local write "高正开关"(w395) -> ()
                n187 = local write "大气压"(TRUE) -> ()
              }
              frame #1 {
                n188 = local write "case"(5.0) -> ()
              }
              frame #2 {
                n189 = Tick Count (ms)() -> (millisecond timer value=w398:u32)
                n190 = local write "起始破膜时间"(w398) -> ()
                n191 = local write "自动破膜"(TRUE) -> ()
                n192 = local write "自动封接"(FALSE) -> ()
                n193 = One Button Dialog(message="已形成G欧封接！" ("消息")) -> ()  [unwired: 1 in, 1 out]
              }
            }
          }
          frame False {
            n194 = flat-sequence {
              frame #0 {
                w402 = FALSE
                n195 = local write "高负开关"(w402) -> ()
                n196 = local write "低正开关"(w402) -> ()
                n197 = local write "高正开关"(w402) -> ()
                n198 = local write "低负开关"(TRUE) -> ()
                n199 = local write "大气压"(w402) -> ()
              }
              frame #1 {
                n200 = local write "case"(4.0) -> ()
              }
              frame #2 {
                n201 = local read "自动封接开始时间"() -> (w408:u32)
                n202 = Tick Count (ms)() -> (millisecond timer value=w409:u32)
                n203 = Subtract(x=w409, y=w408) -> (x-y=w407:u32)
                n204 = Greater?(x=w407, y=u32 200000) -> (0:w405:bool)
                n205 = case shown="真" w405 {
                  frame False {
                  }
                  frame True {
                    n206 = local write "自动封接"(FALSE) -> ()
                    n207 = One Button Dialog(message="自动封接失败！！" ("消息")) -> ()  [unwired: 1 in, 1 out]
                  }
                }
              }
            }
          }
        }
      }
    }
    n208 = case shown="2" "case" {
      tunnel: w280 -> [w438 w458 w480 w504 w528 w541]
      tunnel: w279 -> [w437 w457 w479 w503 w527 w540]
      tunnel: [w438 w440 w471 w498 w520 w538] -> w278
      tunnel: [w437 w448 w472 w497 w521 w537] -> w276
      tunnel: [w435 w439 w463 w487 w511 w535] -> w282
      frame Default {
        w436 = 0.0
        n209 = Bundle(w436, w436) -> (w435:cluster{dbl, dbl})  [unwired: 1 in]
      }
      frame 1 {
        w455 = TRUE
        w456 = FALSE
        n210 = Build Array(w456, w455, w455, w456, w456, w456, w456, w456) -> (w459:bool[])
        n211 = Boolean Array To Number(Boolean array=w459) -> (number=w462:u32)
        n212 = To Unsigned Byte Integer(number=w462) -> (unsigned 8bit integer=w461:u8)
        n213 = call "StartRead.vi"("错误输入（无错误）"=w457, "DevIndex"=w458) -> ("错误输出"=w453:errorcluster, "DevIndex Output"=w454:i32)  [unwired: 8 in]
        n214 = call "SetDioOut.vi"("错误输入（无错误）"=w453, "DioOut"=w461, "DioChanSel"=u8 255, "DevIndex"=w454) -> ("错误输出"=w449:errorcluster, "DevIndex Output"=w450:i32)  [unwired: 6 in]
        n215 = call "GetAiChans.vi"("错误输入（无错误）"=w449, "Num"=u32 1, "ChanSel"=u16 1, "DevIndex"=w450) -> ("错误输出"=w448:errorcluster, "Ai"=w445:sgl[][], "DevIndex Output"=w440:i32)  [unwired: 4 in, 1 out]
        n216 = Index Array(array=w445, index (row)=0, index (col)=0) -> (element=w442:sgl)
        n217 = local read "高正"() -> (w444:sgl)
        n218 = Multiply(x=w442, y=3) -> (x*y=w441:sgl)
        n219 = Bundle(w441, "高正"=w444) -> (w439:cluster{sgl, "高正":sgl})  [unwired: 1 in]
      }
      frame 2 {
        w478 = TRUE
        w477 = FALSE
        n220 = Build Array(w477, w478, w477, w477, w478, w477, w477, w477) -> (w481:bool[])
        n221 = Boolean Array To Number(Boolean array=w481) -> (number=w486:u32)
        n222 = To Unsigned Byte Integer(number=w486) -> (unsigned 8bit integer=w485:u8)
        n223 = call "StartRead.vi"("错误输入（无错误）"=w479, "DevIndex"=w480) -> ("错误输出"=w482:errorcluster, "DevIndex Output"=w483:i32)  [unwired: 8 in]
        n224 = call "SetDioOut.vi"("错误输入（无错误）"=w482, "DioOut"=w485, "DioChanSel"=u8 255, "DevIndex"=w483) -> ("错误输出"=w473:errorcluster, "DevIndex Output"=w474:i32)  [unwired: 6 in]
        n225 = call "GetAiChans.vi"("错误输入（无错误）"=w473, "Num"=u32 1, "ChanSel"=u16 2, "DevIndex"=w474) -> ("错误输出"=w472:errorcluster, "Ai"=w468:sgl[][], "DevIndex Output"=w471:i32)  [unwired: 4 in, 1 out]
        n226 = Unbundle(w473) -> ()  [unwired: 3 out]
        n227 = Index Array(array=w468, index (row)=0, index (col)=0) -> (element=w466:sgl)
        n228 = local read "高负"() -> (w467:sgl)
        n229 = Multiply(x=w466, y=-1.004) -> (x*y=w464:dbl)
        n230 = Bundle(w464, "高负"=w467) -> (w463:cluster{dbl, "高负":sgl})  [unwired: 1 in]
      }
      frame 3 {
        w489 = FALSE
        n231 = Build Array(w489, w489, w489, TRUE, w489, w489, w489, w489) -> (w505:bool[])
        n232 = Boolean Array To Number(Boolean array=w505) -> (number=w510:u32)
        n233 = To Unsigned Byte Integer(number=w510) -> (unsigned 8bit integer=w509:u8)
        n234 = call "StartRead.vi"("错误输入（无错误）"=w503, "DevIndex"=w504) -> ("错误输出"=w506:errorcluster, "DevIndex Output"=w507:i32)  [unwired: 8 in]
        n235 = call "SetDioOut.vi"("错误输入（无错误）"=w506, "DioOut"=w509, "DioChanSel"=u8 255, "DevIndex"=w507) -> ("错误输出"=w499:errorcluster, "DevIndex Output"=w500:i32)  [unwired: 6 in]
        n236 = call "GetAiChans.vi"("错误输入（无错误）"=w499, "Num"=u32 1, "ChanSel"=u16 4, "DevIndex"=w500) -> ("错误输出"=w497:errorcluster, "Ai"=w494:sgl[][], "DevIndex Output"=w498:i32)  [unwired: 4 in, 1 out]
        n237 = Unbundle(w499) -> ()  [unwired: 3 out]
        n238 = Index Array(array=w494, index (row)=0, index (col)=0) -> (element=w492:sgl)
        n239 = local read "低正"() -> (w493:sgl)
        n240 = Divide(x=w492, y=2.564) -> (x/y=w490:dbl)
        n241 = Bundle(w490, "低正"=w493) -> (w487:cluster{dbl, "低正":sgl})  [unwired: 1 in]
      }
      frame 4 {
        w512 = FALSE
        n242 = call "StartRead.vi"("错误输入（无错误）"=w527, "DevIndex"=w528) -> ("错误输出"=w530:errorcluster, "DevIndex Output"=w531:i32)  [unwired: 8 in]
        n243 = local read "低负"() -> (w516:sgl)
        n244 = Build Array(w512, w512, w512, w512, w512, TRUE, w512, w512) -> (w529:bool[])
        n245 = Boolean Array To Number(Boolean array=w529) -> (number=w534:u32)
        n246 = To Unsigned Byte Integer(number=w534) -> (unsigned 8bit integer=w533:u8)
        n247 = call "SetDioOut.vi"("错误输入（无错误）"=w530, "DioOut"=w533, "DioChanSel"=u8 255, "DevIndex"=w531) -> ("错误输出"=w522:errorcluster, "DevIndex Output"=w523:i32)  [unwired: 6 in]
        n248 = Unbundle(w522) -> ()  [unwired: 3 out]
        n249 = call "GetAiChans.vi"("错误输入（无错误）"=w522, "Num"=u32 1, "ChanSel"=u16 8, "DevIndex"=w523) -> ("错误输出"=w521:errorcluster, "Ai"=w517:sgl[][], "DevIndex Output"=w520:i32)  [unwired: 4 in, 1 out]
        n250 = Index Array(array=w517, index (row)=0, index (col)=0) -> (element=w515:sgl)
        n251 = Divide(x=w515, y=-2.294) -> (x/y=w513:dbl)
        n252 = Bundle(w513, "低负"=w516) -> (w511:cluster{dbl, "低负":sgl})  [unwired: 1 in]
      }
      frame 5 {
        w536 = 0.0
        (unwired) TRUE
        w539 = FALSE
        n253 = call "StartRead.vi"("错误输入（无错误）"=w540, "DevIndex"=w541) -> ("错误输出"=w543:errorcluster, "DevIndex Output"=w544:i32)  [unwired: 8 in]
        n254 = Build Array(w539, w539, w539, w539, w539, w539, w539, w539) -> (w542:bool[])
        n255 = Boolean Array To Number(Boolean array=w542) -> (number=w547:u32)
        n256 = To Unsigned Byte Integer(number=w547) -> (unsigned 8bit integer=w546:u8)
        n257 = call "SetDioOut.vi"("错误输入（无错误）"=w543, "DioOut"=w546, "DioChanSel"=u8 255, "DevIndex"=w544) -> ("错误输出"=w537:errorcluster, "DevIndex Output"=w538:i32)  [unwired: 6 in]
        n258 = Unbundle(w537) -> ()  [unwired: 3 out]
        n259 = Bundle(w536, w536) -> (w535:cluster{dbl, dbl})  [unwired: 1 in]
      }
    }
    "输出气压波形图表" <- w282
    n260 = Unbundle(w282) -> (→"测量值":dbl, "高正"=→"给定值":dbl)
    n261 = case shown="真" "自动破膜" {
      frame False {
      }
      frame True {
        n262 = local read "阻值数组"() -> (w330:dbl[])
        n263 = Index Array(array=w330, index=0 ("索引")) -> (element=w326:dbl)
        n264 = Less?(x=500.0 ("y"), y=w326) -> (x < y?=w328:bool)
        n265 = case shown="真" w328 {
          frame False {
            n266 = local write "自动破膜"(FALSE) -> ()
            n267 = One Button Dialog(message="恭喜你，成功破膜" ("消息")) -> ()  [unwired: 1 in, 1 out]
          }
          frame True {
            n268 = case shown="\"200ms\", 默认" "枚举" {
              tunnel: [200.0 1000.0 500.0] -> w333
              frame "200ms", Default {
              }
              frame "1000ms" {
              }
              frame "500ms" {
              }
            }
            n269 = Tick Count (ms)() -> (millisecond timer value=w335:u32)
            n270 = local read "起始破膜时间"() -> (w338:u32)
            n271 = Subtract(x=w335, y=w338) -> (x-y=w336:u32)
            n272 = Greater?(x=w333, y=w336) -> (0:w337:bool)
            n273 = case shown="真" w337 {
              frame False {
                n274 = flat-sequence {
                  frame #0 {
                    w344 = FALSE
                    n275 = local write "高负开关"(w344) -> ()
                    n276 = local write "低正开关"(w344) -> ()
                    n277 = local write "高正开关"(w344) -> ()
                    n278 = local write "低负开关"(w344) -> ()
                    n279 = local write "大气压"(TRUE) -> ()
                    n280 = local write "case"(5.0) -> ()
                  }
                  frame #1 {
                    n281 = local write "自动破膜"(FALSE ("自动破膜")) -> ()
                  }
                }
              }
              frame True {
                n282 = flat-sequence {
                  frame #0 {
                    w348 = FALSE
                    n283 = local write "高负开关"(TRUE) -> ()
                    n284 = local write "低正开关"(w348) -> ()
                    n285 = local write "高正开关"(w348) -> ()
                    n286 = local write "低负开关"(w348) -> ()
                    n287 = local write "大气压"(w348) -> ()
                    n288 = local write "case"(2.0) -> ()
                  }
                  frame #1 {
                    n289 = local write "高负"(-5.0) -> ()
                  }
                }
              }
            }
          }
        }
      }
    }
  }
  n290 = while {
    tunnel: w143 -> [w557]
    tunnel: [w556] -> w75
    tunnel: w41 -> [w555]
    tunnel: w40 -> [w554]
    stop <- w552 stop-if-true
    # "电流信号循环"
    n291 = Dequeue Element(queue=w555, timeout in ms (-1)=1 ("超时毫秒(-1)"), error in (no error)=w554) -> (error out=w550:errorcluster)  [unwired: 3 out]
    n292 = Unbundle By Name(w550) -> ("status"=w552:bool)
    n293 = flat-sequence {
      tunnel: w557 -> [w578]
      tunnel: [w578] -> w549
      tunnel: [w566] -> w548
      tunnel: [w586] -> w559
      tunnel: [w601] -> w558
      tunnel: w549 -> [w587]
      tunnel: w548 -> [w601]
      tunnel: [w623] -> w563
      tunnel: [w608] -> w562
      tunnel: w559 -> [w603]
      tunnel: w558 -> [w619]
      tunnel: w563 -> [w697]
      tunnel: w562 -> [w698]
      tunnel: w557 -> [w699]
      tunnel: [w696] -> w561
      tunnel: [w688] -> w560
      tunnel: [w741] -> w556
      tunnel: w561 -> [w741]
      tunnel: w560 -> [w739]
      frame #0 {
        n294 = case shown="假" "控制箱刺激ON\n/放大器刺激" {
          tunnel: [0.0 ("data") 5.0 ("data")] -> w575
          frame False {
          }
          frame True {
          }
        }
        n295 = call-poly <vilib>:"DAQmx Create Virtual Channel.vi"("physical channels"=tag "Dev2/ao1") -> ("task out"=w571:refnum<k21>, "error out"=w572:errorcluster)  [unwired: 13 in]
        n296 = call <vilib>:"DAQmx Start Task.vi"("task/channels in"=w571, "error in"=w572) -> ("task out"=w570:refnum<k21>, "error out"=w569:errorcluster)  [unwired: 12 in]
        n297 = call-poly <vilib>:"DAQmx Write.vi"("task/channels in"=w570, "data"=w575, "error in"=w569) -> ("task out"=w568:refnum<k21>, "error out"=w567:errorcluster)  [unwired: 10 in, 1 out]
        n298 = call <vilib>:"DAQmx Stop Task.vi"("task/channels in"=w568, "error in"=w567) -> ("task out"=w574:refnum<k21>, "error out"=w573:errorcluster)  [unwired: 12 in]
        n299 = call <vilib>:"DAQmx Clear Task.vi"("task in"=w574, "error in"=w573) -> ("error out"=w566:errorcluster)  [unwired: 13 in]
      }
      frame #1 {
        n300 = Unbundle By Name(w587) -> ("amplitude"=w593:dbl, "frequency"=w592:dbl, "Fs"=w594:dbl, "Averaging"=w595:i32)
        n301 = Multiply(x=w594, y=w595) -> (x*y=w590:dbl)
        n302 = Multiply(x="钳制电位", y="Holding Voltage") -> (x*y=w583:dbl)
        n303 = Divide(x=w590, y=w592) -> (x/y=w591:dbl)
        n304 = Divide(x=w593, y=2.0) -> (x/y=w597:dbl)
        n305 = Add(x=w583, y=0.5) -> (x+y=w581:dbl)
        "x*y" <- w581
        n306 = Divide(x=w581, y=1000.0) -> (x/y=w598:dbl)
        n307 = Add(x=w598, y=w597) -> (x+y=w588:dbl)
        n308 = Bundle("Fs"=w594, w591) -> (w596:cluster{"Fs":dbl, dbl})  [unwired: 1 in]
        n309 = call <vilib>:"Basic Function Generator.vi"("offset"=w588, "sampling info"=w596, "signal type"=T10."Square Wave", "amplitude"=w597, "frequency"=w592) -> ("signal out"=w586:waveform(dbl))  [unwired: 4 in, 2 out]
      }
      frame #2 {
        w651 = 10178 items=["有限采样"=10178, "连续采样"=10123, "硬件定时单点"=12522] ("sample mode")
        w652 = tag "OnboardClock" ("source")
        w644 = 10178 items=["有限采样"=10178, "连续采样"=10123, "硬件定时单点"=12522] ("sample mode")
        # "必须要有触发"
        # "This version of StimRecord is for the NI DAQ used in conjunction with the MultiClamp 700b"
        # "multiclamp放大器自己参数"
        # "in V"
        # "in nA"
        n310 = case shown="0, 默认" "电压钳/电流钳" {
          tunnel: [50.0 ("y") 2500000000.0 ("y")] -> w620
          tunnel: [2000.0 ("y") 0.1 ("y")] -> w621
          frame 0, Default {
          }
          frame 1 {
          }
        }
        n311 = Multiply(x=w603, y=w620) -> (x*y=w638:waveform(dbl))
        n312 = call-poly <vilib>:"Waveform Duration.vi"("waveform in"=w603) -> ("duration"=w639:dbl)  [unwired: 8 in, 2 out]
        n313 = Unbundle By Name(w638) -> ("Y"=w607:dbl[], "dt"=w637:dbl)
        n314 = for {
          tunnel: [w666] -> w606 mode=indexing
          tunnel: w607 -> [w660] mode=indexing
          w661 = 10.0 ("t")
          w664 = -10.0 ("t")
          n315 = Greater?(x=w664, y=w660) -> (0:w665:bool)
          n316 = Select(t=w664, s=w665, f=w660) -> (s? t:f=w662:dbl)
          n317 = Less?(x=w661, y=w662) -> (x < y?=w663:bool)
          n318 = Select(t=w661, s=w663, f=w662) -> (s? t:f=w666:dbl)
        }
        n319 = Multiply(x=w639, y=2.0) -> (x*y=w640:dbl)
        n320 = Add(x=w640, y=5.0) -> (x+y=w610:dbl)
        n321 = call-poly <vilib>:"DAQmx Create Virtual Channel.vi"("physical channels"=tag "Dev2/ai0", "error in"=w619) -> ("task out"=w643:refnum<k21>, "error out"=w642:errorcluster)  [unwired: 12 in]
        n322 = call-poly <vilib>:"DAQmx Create Virtual Channel.vi"("physical channels"=tag "Dev2/ao0", "error in"=w619) -> ("task out"=w633:refnum<k21>, "error out"=w632:errorcluster)  [unwired: 12 in]
        n323 = Reciprocal(x=w637) -> (1/x=w645:dbl)
        n324 = Array Size(array=w607) -> (size(s)=w659:i32)
        n325 = call-poly <vilib>:"DAQmx Timing.vi"("task/channels in"=w633, "sample mode"=w651, "samples per channel"=w659, "rate"=w645, "source"=w652, "error in"=w632) -> ("task out"=w618:refnum<k21>, "error out"=w616:errorcluster)  [unwired: 8 in]
        n326 = Bundle By Name(cluster=w638, "Y"=w606) -> (w602:waveform(dbl))
        n327 = call-poly <vilib>:"DAQmx Timing.vi"("task/channels in"=w643, "sample mode"=w644, "samples per channel"=w659, "rate"=w645, "source"=w652, "error in"=w642) -> ("task out"=w647:refnum<k21>, "error out"=w648:errorcluster)  [unwired: 8 in]
        n328 = call-poly <vilib>:"DAQmx Trigger.vi"("task/channels in"=w618, "source"=tag "/Dev2/ai/StartTrigger", "error in"=w616) -> ("task out"=w617:refnum<k21>, "error out"=w615:errorcluster)  [unwired: 11 in]
        n329 = call-poly <vilib>:"DAQmx Write.vi"("task/channels in"=w617, "auto start"=FALSE, "data"=w602, "timeout"=w610, "error in"=w615) -> ("task out"=w636:refnum<k21>, "error out"=w656:errorcluster)  [unwired: 8 in, 1 out]
        n330 = property class="DAQmx定时" props=["SampClk.Rate"](reference=w647, error in=w648) -> (reference out=w649:refnum<k21>)  [unwired: 2 out]
        n331 = call <vilib>:"DAQmx Start Task.vi"("task/channels in"=w636, "error in"=w656) -> ("task out"=w653:refnum<k21>, "error out"=w655:errorcluster)  [unwired: 12 in]
        n332 = call <vilib>:"DAQmx Start Task.vi"("task/channels in"=w649, "error in"=w655) -> ("task out"=w628:refnum<k21>, "error out"=w629:errorcluster)  [unwired: 12 in]
        n333 = call-poly <vilib>:"DAQmx Read.vi"("task/channels in"=w628, "number of samples per channel"=w659, "timeout"=w610, "error in"=w629) -> ("task out"=w614:refnum<k21>, "data"=w641:waveform(dbl), "error out"=w612:errorcluster)  [unwired: 9 in]
        n334 = call <vilib>:"DAQmx Is Task Done.vi"("task/channels in"=w653, "error in"=w655) -> ("task out"=w654:refnum<k21>, "error out"=w657:errorcluster)  [unwired: 11 in, 1 out]
        n335 = call <vilib>:"DAQmx Wait Until Done.vi"("task/channels in"=w654, "timeout (sec)"=w610, "error in"=w657) -> ("task out"=w634:refnum<k21>, "error out"=w635:errorcluster)  [unwired: 11 in]
        n336 = call <vilib>:"DAQmx Wait Until Done.vi"("task/channels in"=w614, "timeout (sec)"=w610, "error in"=w612) -> ("task out"=w613:refnum<k21>, "error out"=w611:errorcluster)  [unwired: 11 in]
        n337 = call <vilib>:"DAQmx Stop Task.vi"("task/channels in"=w634, "error in"=w635) -> ("task out"=w631:refnum<k21>, "error out"=w630:errorcluster)  [unwired: 12 in]
        n338 = Multiply(x=w641, y=w621) -> (x*y=w608:waveform(dbl))
        "电流信号波形图" <- w608
        n339 = call <vilib>:"DAQmx Stop Task.vi"("task/channels in"=w613, "error in"=w611) -> ("task out"=w626:refnum<k21>, "error out"=w627:errorcluster)  [unwired: 12 in]
        n340 = call <vilib>:"DAQmx Clear Task.vi"("task in"=w631, "error in"=w630) -> ("error out"=w658:errorcluster)  [unwired: 13 in]
        n341 = call <vilib>:"DAQmx Clear Task.vi"("task in"=w626, "error in"=w627) -> ("error out"=w625:errorcluster)  [unwired: 13 in]
        n342 = Merge Errors(w658, w625) -> (w623:errorcluster)
        n343 = Build Array(w638, w608) -> ()  [unwired: 1 out]
      }
      frame #3 {
        # "数据读取错误"
        # "阻值读取异常处理"
        # "单位换算不明白"
        # "阻值处理"
        # "Convert Volts/pA into MOhms"
        n344 = call "Filter"("error in (no error)"=w697, "Signal"=w698) -> ("error out"=w700:errorcluster, "Filtered Signal"=w692:dynamicdata)  [unwired: 8 in]
        n345 = call "单频测量"("Signals"=w692) -> ("Frequency"=w691:dynamicdata)  [unwired: 9 in, 1 out]
        n346 = Unbundle By Name(w699) -> ("Fs"=w713:dbl, "frequency"=w712:dbl, "Proportion"=w705:dbl)
        n347 = Unbundle By Name(w699) -> ("Averaging"=w711:i32)
        n348 = call "Convert from Dynamic Data"("Dynamic Data Type"=w692) -> ("Array"=w703:dbl[])  [unwired: 3 in]
        n349 = call "从动态数据转换"("Dynamic Data Type"=w691) -> ("Array"=w690:dbl[])  [unwired: 3 in]
        n350 = call-poly <vilib>:"Mean.vi"("X"=w690) -> ("mean"=w687:dbl)  [unwired: 1 out]
        n351 = Divide(x=w713, y=w712) -> (x/y=w716:dbl)
        n352 = Reshape Array(w703, w711, w716) -> (w715:dbl[][])
        n353 = call-poly <vilib>:"Mean.vi"("X"=w703) -> ("mean"=w704:dbl)  [unwired: 1 out]
        n354 = for {
          N: w711 -> [_]
          tunnel: w715 -> [w727] mode=indexing
          tunnel: w700 -> [w734]
          shift-right: [w735] -> w714
          shift-left: dbl[] [] -> [w736]
          tunnel: [w722] -> w710
          tunnel: [w734] -> w696
          tunnel: w705 -> [w726]
          # "不是整个电流的均值"
          # "波形后半段"
          # "波形前半段"
          n355 = Array Size(array=w727) -> (size(s)=w724:i32)
          n356 = Subtract(x=1.0, y=w726) -> (x-y=w729:dbl)
          n357 = Divide(x=w724, y=2) -> (x/y=w731:dbl)
          n358 = Multiply(x=w731, y=w729) -> (x*y=w728:dbl)
          n359 = Split 1D Array(array=w727, index=w731) -> (first subarray=w723:dbl[], second subarray=w732:dbl[])
          n360 = Split 1D Array(array=w723, index=w728) -> (second subarray=w719:dbl[])  [unwired: 1 out]
          n361 = Split 1D Array(array=w732, index=w728) -> (second subarray=w720:dbl[])  [unwired: 1 out]
          n362 = call-poly <vilib>:"Mean.vi"("X"=w719) -> ("mean"=w721:dbl)  [unwired: 1 out]
          n363 = call-poly <vilib>:"Mean.vi"("X"=w720) -> ("mean"=w722:dbl)  [unwired: 1 out]
          n364 = Subtract(x=w721, y=w722) -> (x-y=w725:dbl)
          n365 = Build Array (concatenate)(w736, w725) -> (w735:dbl[])
        }
        "Negative Peak" <- w710
        n366 = Subtract(x=w687, y=sgl 20.0) -> (x-y=w685:dbl)
        n367 = Array Max & Min(array=w703) -> (min value=w702:dbl)  [unwired: 3 out]
        n368 = Absolute Value(x=w685) -> (abs(x)=w684:dbl)
        n369 = Greater?(x=w684, y=0.05) -> (0:w678:bool)
        "！" <- w678
        n370 = Subtract(x=w704, y=w702) -> (x-y=w701:dbl)
        n371 = Unbundle By Name(w699) -> ("amplitude"=w708:dbl)
        n372 = Multiply(x=w708, y=1000000.0) -> (x*y=w695:dbl)
        n373 = Divide(x=w695, y=w701) -> (x/y=→"电阻值":dbl)
        n374 = call-poly <vilib>:"Mean.vi"("X"=w714) -> ("mean"=w709:dbl)  [unwired: 1 out]
        n375 = local read "Resistance(MΩ)"() -> (w681:dbl)
        n376 = Divide(x=w695, y=w709) -> (x/y=w694:dbl)
        n377 = Multiply(x=w694, y=2.0) -> (x*y=w693:dbl)
        n378 = local read "阻值数组"() -> (w689:dbl[])
        n379 = Less?(x=w681, y=100.0) -> (x < y?=w679:bool)
        n380 = And(x=w679, y=w678) -> (x .and. y?=w677:bool)
        n381 = case shown="假" w677 {
          tunnel: w681 -> [_ w718]
          tunnel: w693 -> [w717 _]
          tunnel: [w717 w718] -> w676
          frame False {
          }
          frame True {
          }
        }
        n382 = In Range and Coerce(upper limit=10000.0 ("上限"), x=w676, lower limit=0.0 ("下限")) -> (coerced(x)=w671:dbl)  [unwired: 1 out]
        "阻值波形图表" <- w671
        "Resistance(MΩ)" <- w671
        n383 = Insert Into Array(array=w689, index=0 ("索引"), new element=w671) -> (w688:dbl[])
        n384 = local write "阻值数组"(w688) -> ()
      }
      frame #4 {
        n385 = Array Size(array=w739) -> (size(s)=w738:i32)
        n386 = Greater?(x=w738, y=10) -> (0:w737:bool)
        n387 = case shown="真" w737 {
          tunnel: w739 -> [_ w744]
          frame False {
          }
          frame True {
            n388 = Delete From Array(array=w744, length=1 ("长度")) -> (array with subset deleted=w742:dbl[])  [unwired: 1 in, 1 out]
            n389 = local write "阻值数组"(w742) -> ()
          }
        }
      }
    }
    n390 = case shown="真" "入液阻值校准" {
      frame False {
      }
      frame True {
        n391 = flat-sequence {
          frame #0 {
            n392 = local read "Resistance(MΩ)"() -> (→"校准的入液阻值":dbl)
          }
          frame #1 {
            n393 = local write "入液阻值校准"(FALSE) -> ()
          }
        }
      }
    }
  }
  n394 = VISA Close(VISA resource name=w43, error in (no error)=w42) -> ()  [unwired: 1 out]
  n395 = call "IMAQ Create"("Image Name"="") -> ("New Image"=w1:T4)  [unwired: 4 in, 1 out]
  n396 = call "IMAQ Create"("Image Name"="针尖图像处理") -> ("New Image"=w78:T4)  [unwired: 4 in, 1 out]
  n397 = call "IMAQ Create"("Image Name"="二值化") -> ("New Image"=w77:T4)  [unwired: 4 in, 1 out]
  n398 = call "IMAQ Create"("Image Name"="镜像") -> ("New Image"=w20:T4)  [unwired: 4 in, 1 out]
  n399 = call "IMAQ Create"("Image Name"="", "Image Type"=w11) -> ("New Image"=w14:T4)  [unwired: 3 in, 1 out]
  n400 = call "IMAQ ReadFile 2"("File Path"=path "C:/Users/MPQ/Desktop/2.bmp", "Image"=w14) -> ("Image Out"=w10:T4)  [unwired: 5 in, 4 out]
  n401 = call "IMAQ Create"("Image Name"="上一张") -> ("New Image"=w22:T4)  [unwired: 4 in, 1 out]
  n402 = call "IMAQ Create"("Image Name"="") -> ("New Image"=w8:T4)  [unwired: 4 in, 1 out]
  n403 = call "IMAQ ExtractSingleColorPlane"("Image Dst"=w8, "Image Src"=w10) -> ()  [unwired: 8 in, 2 out]
  n404 = call "IMAQ Create"("Image Name"="", "Image Type"=w30) -> ("New Image"=w27:T4)  [unwired: 3 in, 1 out]
  n405 = call "IMAQ Create"("Image Name"="", "Image Type"=w28) -> ("New Image"=w26:T4)  [unwired: 3 in, 1 out]
  n406 = call "IMAQ Create"("Image Name"="unet裁剪") -> ("New Image"=w48:T4)  [unwired: 4 in, 1 out]
  n407 = call "IMAQ Create"("Image Name"="mask图像") -> ("New Image"=w46:T4)  [unwired: 4 in, 1 out]
  n408 = while {
    tunnel: w153 -> [w794]
    tunnel: w151 -> [w793]
    tunnel: [w770] -> w146
    shift-right: [w791] -> _
    shift-left: _ -> [w790]
    tunnel: w144 -> [w789]
    tunnel: [w788] -> w141
    tunnel: w140 -> [w787]
    tunnel: [w786] -> w139
    tunnel: w138 -> [w785]
    tunnel: w41 -> [w784]
    tunnel: [w781] -> w136
    shift-right: [w780] -> w135
    shift-left: w40 -> [w779]
    tunnel: w81 -> [w778]
    tunnel: w78 -> [w777]
    tunnel: w77 -> [w776]
    tunnel: w48 -> [w769]
    tunnel: w46 -> [w751]
    tunnel: w22 -> [_]
    tunnel: w20 -> [w767]
    tunnel: w16 -> [w766]
    tunnel: w3 -> [w750]
    tunnel: w1 -> [w749]
    tunnel: [w746] -> w142
    stop <- "停止" stop-if-true
    w759 = 0 items=["Red", "Green", "Blue", "Hue", "Saturation", "Luminance", "Value", "Intensity"] ("Color Plane")
    # "图像检测"
    # "图像处理循环"
    n409 = Tick Count (ms)() -> (millisecond timer value=w791:u32)
    n410 = call <vilib>:"IMAQdx Grab2.vi"("error in"=w787, "Image In"=w793, "Session In"=w794) -> ("error out"=w786:errorcluster, "Image Out"=w758:T4, "Session Out"=w770:T6)  [unwired: 5 in, 1 out]
    n411 = Subtract(x=w791, y=w790) -> (x-y=→"循环时间":u32)
    n412 = call "IMAQ ExtractSingleColorPlane"("Color Plane"=w759, "error in (no error)"=w785, "Image Dst"=w789, "Image Src"=w758) -> ("error out"=w788:errorcluster, "Image Dst Out"=w746:T4)  [unwired: 6 in]
    n413 = Enqueue Element(queue=w784, element="停止", timeout in ms (-1)=1 ("超时毫秒(-1)"), error in (no error)=w779) -> (queue out=w781:refnum<queue>, error out=w780:errorcluster)  [unwired: 1 out]
    n414 = local read "针尖移动 2"() -> (w763:bool)
    n415 = local read "针尖细对焦"() -> (w765:bool)
    n416 = local read "针尖移动"() -> (w764:bool)
    n417 = local read "升Z轴找针"() -> (w762:bool)
    n418 = Or(x=w765, y=w764) -> (x .or. y?=w761:bool)
    n419 = Or(x=w761, y="针尖模板匹配") -> (x .or. y?=w760:bool)
    n420 = Compound Arithmetic op=OR("针尖模板匹配", w765, w762, w764, w763) -> ()  [unwired: 1 out]
    n421 = case shown="真" TRUE {
      tunnel: w778 -> [_ w1017]
      tunnel: w746 -> [w1006 w1020]
      tunnel: [FALSE w1053] -> w773
      tunnel: [w1006 w1019] -> w753
      tunnel: w766 -> [_ w1015]
      tunnel: w760 -> [_ _]
      tunnel: "针尖模板匹配" -> [_ w1008]
      frame False {
      }
      frame True {
        w1022 = u32 1 items=["Frame", "Fill", "Highlight"] ("Drawing Mode (Frame)")
        w1025 = 10.0 ("y")
        w1047 = u16 0 items=["All", "Shift Information", "Rotation Information"] ("Learn Mode")
        # "目标和针尖坐标获取"
        # "模板针尖偏移量"
        # "是否匹配到"
        # "模板匹配针尖"
        n422 = case shown="假" w1008 {
          tunnel: [w1057 w1058] -> w1016
          tunnel: w1017 -> [_ w1058]
          tunnel: w1015 -> [w1057 _]
          frame False {
          }
          frame True {
          }
        }
        n423 = call "IMAQ Setup Match Pattern 2"("Minimum Contrast"="Minimum Contrast", "Match Mode"="Match Mode") -> ("Match Pattern Setup Data"=w1051:string)  [unwired: 8 in, 1 out]
        n424 = call "IMAQ Setup Learn Pattern 2"("Learn Mode"=w1047) -> ("Learn Pattern Setup Data"=w1046:string)  [unwired: 9 in, 1 out]
        n425 = call "IMAQ Learn Pattern 2"("Learn Pattern Setup Data"=w1046, "Image"=w1016) -> ("Template Image Out"=w1043:T4)  [unwired: 8 in, 1 out]
        n426 = call "IMAQ Match Pattern 2"("Minimum Match Score"="Minimum Match Score", "Number of Matches Requested"="Number of Matches Requested", "Match Pattern Setup Data"=w1051, "Template Image"=w1043, "Image"=w1020) -> ("Number of Matches"=w1044:i32, "Matches"=w1041:T1)  [unwired: 4 in, 1 out]
        "Number of Matches" <- w1044
        "Matches 2" <- w1041
        n427 = Equal?(x=w1044, y=0) -> ()  [unwired: 1 out]
        n428 = local read "升Z轴找针"() -> (w1010:bool)
        n429 = case shown="假" w1010 {
          tunnel: [sgl 650.0 ("y") "模板分数"] -> w1009
          frame False {
          }
          frame True {
          }
        }
        n430 = Index Array(array=w1041, index=0 ("索引")) -> (element=w1039:T11)
        n431 = Index Array(array=w1041, index=0 ("索引")) -> (element=w1024:T11)
        n432 = Unbundle(w1039) -> ("Score"=w1038:sgl)  [unwired: 4 out]
        n433 = Less?(x=w1038, y=w1009) -> (x < y?=w1053:bool)
        n434 = Unbundle(w1024) -> ("Position"=w1023:cluster{"x":sgl, "y":sgl})  [unwired: 4 out]
        n435 = Cluster To Array(cluster=w1023) -> (array=w1011:sgl[])
        n436 = Equal?(x=w1011, y=sgl[] [0.0, 0.0]) -> (x = y?=w1013:bool[])
        n437 = And Array Elements(Boolean array=w1013) -> (logical AND=w1012:bool)
        n438 = case shown="假" w1012 {
          tunnel: w1011 -> [w1056 _]
          frame False {
            "针尖坐标" <- w1056
          }
          frame True {
          }
        }
        n439 = Unbundle(w1023) -> ("x"=w1034:sgl, "y"=w1037:sgl)
        n440 = Add(x=w1034, y=sgl 0.0) -> (x+y=w1036:sgl)
        n441 = Subtract(x=w1037, y=w1025) -> (x-y=w1028:dbl)
        n442 = Add(x=w1037, y=w1025) -> (x+y=w1027:dbl)
        n443 = Subtract(x=w1036, y=w1025) -> (x-y=w1026:dbl)
        n444 = Add(x=w1036, y=w1025) -> (x+y=w1029:dbl)
        n445 = To Long Integer(number=w1028) -> (32bit integer=w1031:i32)
        n446 = To Long Integer(number=w1027) -> (32bit integer=w1032:i32)
        n447 = To Long Integer(number=w1026) -> (32bit integer=w1030:i32)
        n448 = To Long Integer(number=w1029) -> (32bit integer=w1033:i32)
        n449 = Bundle(w1030, w1031, w1033, w1032) -> (w1021:cluster{i32, i32, i32, i32})  [unwired: 1 in]
        n450 = call "IMAQ Overlay Oval"("Color"=u32 6618880, "Drawing Mode (Frame)"=w1022, "Bounding Rectangle"=w1021, "Image"=w1020) -> ("Image Out"=w1019:T4)  [unwired: 6 in, 1 out]
      }
    }
    "没匹配到？" <- w773
    n451 = case shown="真" "目标细胞位置" {
      tunnel: [w795 w805] -> w754
      tunnel: w753 -> [w795 w804]
      frame False {
      }
      frame True {
        w799 = 0 ("索引")
        n452 = local read "目标坐标"() -> (w803:i32[])
        n453 = Index Array(array=w803, index=w799) -> (element=w801:i32)
        n454 = Index Array(array=w803, index=1 ("索引")) -> (element=w800:i32)
        n455 = Equal?(x=w801, y=w799) -> (x = y?=w798:bool)
        n456 = Equal?(x=w800, y=w799) -> (x = y?=w797:bool)
        n457 = And(x=w798, y=w797) -> (x .and. y?=w796:bool)
        n458 = case shown="假" w796 {
          tunnel: [w819 w822] -> w805
          tunnel: w804 -> [w818 w822]
          tunnel: w800 -> [w807 _]
          tunnel: w801 -> [w806 _]
          frame False {
            w809 = 10 ("y")
            w820 = u32 1 items=["Frame", "Fill"] ("Drawing Mode (Frame)")
            n459 = Subtract(x=w806, y=w809) -> (x-y=w810:i32)
            n460 = Add(x=w806, y=w809) -> (x+y=w813:i32)
            n461 = Subtract(x=w807, y=w809) -> (x-y=w812:i32)
            n462 = Add(x=w807, y=w809) -> (x+y=w811:i32)
            n463 = To Long Integer(number=w810) -> (32bit integer=w814:i32)
            n464 = To Long Integer(number=w813) -> (32bit integer=w817:i32)
            n465 = To Long Integer(number=w812) -> (32bit integer=w815:i32)
            n466 = To Long Integer(number=w811) -> (32bit integer=w816:i32)
            n467 = Bundle(w814, w815, w817, w816) -> (w808:cluster{i32, i32, i32, i32})  [unwired: 1 in]
            n468 = call "IMAQ Overlay Oval"("Color"=u32 16711680, "Drawing Mode (Frame)"=w820, "Bounding Rectangle"=w808, "Image"=w818) -> ("Image Out"=w819:T4)  [unwired: 6 in, 1 out]
          }
          frame True {
          }
        }
      }
    }
    "Image" <- w754
    n469 = local read "针尖细对焦"() -> (w774:bool)
    n470 = local read "针尖粗对焦"() -> (w775:bool)
    n471 = local read "自动扫描"() -> (w772:bool)
    n472 = Or(x=w775, y=w774) -> (x .or. y?=w771:bool)
    n473 = Or(x=w772, y=w771) -> ()  [unwired: 1 out]
    n474 = case shown="真" "二值化" {
      tunnel: [0.0 ("Right") w972] -> _
      tunnel: w753 -> [_ w960]
      tunnel: w777 -> [_ w1003]
      tunnel: w776 -> [_ w1002]
      tunnel: w767 -> [_ w987]
      tunnel: w750 -> [_ w961]
      tunnel: w749 -> [_ w962]
      frame False {
      }
      frame True {
        w988 = u32 0 items=["Horizontal", "Vertical", "Central", "1st Diagonal", "2nd Diagonal"] ("Type of Symmetry")
        # "目标标定"
        n475 = call "IMAQ Subtract"("Image Src A"=w961, "Image Dst"=w962, "Image Src B"=w960) -> ("Image Dst Out"=w964:T4)  [unwired: 4 in, 1 out]
        n476 = call "IMAQ LowPass"("Image Src"=w964) -> ("Image Dst Out"=w963:T4)  [unwired: 6 in, 1 out]
        n477 = call "IMAQ Threshold"("Range"="Range", "Image Dst"=w1002, "Image Src"=w963) -> ("Image Dst Out"=w1004:T4)  [unwired: 7 in, 1 out]
        n478 = call "IMAQ Copy"("Image Dst"=w1003, "Image Src"=w1004) -> ("Image Dst Out"=w969:T4)  [unwired: 4 in, 1 out]
        n479 = call "IMAQ Morphology"("Operation"="Operation", "Image Src"=w969) -> ("Image Dst Out"=w971:T4)  [unwired: 8 in, 1 out]
        n480 = call "IMAQ Convex Hull"("Image Src"=w971) -> ("Image Dst Out"=w970:T4)  [unwired: 9 in, 1 out]
        n481 = call "IMAQ FillHole"("Image Src"=w970) -> ("Image Dst Out"=w968:T4)  [unwired: 5 in, 1 out]
        n482 = call "IMAQ RemoveParticle"("Number of Erosion"="Number of Erosion", "Image Src"=w968) -> ("Image Dst Out"=w967:T4)  [unwired: 8 in, 1 out]
        n483 = call "IMAQ Clear Overlay"("Image"=w967) -> ("Image Out"=w980:T4)  [unwired: 9 in, 1 out]
        n484 = call "IMAQ ImageToArray"("Image"=w980) -> ("Image Pixels (U8)"=w979:u8[][])  [unwired: 3 in, 4 out]
        n485 = Transpose Matrix(1:w979) -> (0:w989:dbl[][])
        n486 = call "IMAQ ArrayToImage"("Image Pixels (U8)"=w989, "Image"=w987) -> ("Image Out"=w978:T4)  [unwired: 8 in, 1 out]
        n487 = call "IMAQ Symmetry"("Type of Symmetry"=w988, "Image Src"=w978) -> ("Image Dst Out"=w976:T4)  [unwired: 3 in, 1 out]
        "二值化" <- w976
        n488 = call "IMAQ Particle Analysis"("Pixel Measurements"="Pixel Measurements", "Image"=w976) -> ("Particle Measurements (Pixels)"=w990:dbl[][])  [unwired: 4 in, 5 out]
        "Particle Measurements (Pixels)" <- w990
        n489 = call "IMAQ Particle Analysis"("Pixel Measurements"="Pixel Measurements 2", "Image"=w976) -> ("Particle Measurements (Pixels)"=w974:dbl[][])  [unwired: 4 in, 5 out]
        "Particle Measurements (Pixels) 2" <- w974
        n490 = Array Max & Min(array=w990) -> (min value=w982:dbl)  [unwired: 3 out]
        n491 = Subtract(x=3072.0, y=w982) -> (x-y=w972:dbl)
        "Right" <- w972
        n492 = Array Max & Min(array=w974) -> (max value=w986:dbl, min value=w985:dbl)  [unwired: 2 out]
        n493 = Add(x=w986, y=w985) -> (x+y=w984:dbl)
        n494 = Greater?(x=w972, y=500.0) -> (0:w995:bool)
        n495 = Divide(x=w984, y=2.0) -> (x/y=w973:dbl)
        "startY" <- w973
        n496 = Greater?(x=w973, y=300.0) -> (0:w1001:bool)
        n497 = Less?(x=w973, y=1700.0) -> (x < y?=w1000:bool)
        n498 = Less?(x=w972, y=2500.0) -> (x < y?=w996:bool)
        n499 = And(x=w1001, y=w1000) -> (x .and. y?=w993:bool)
        n500 = And(x=w995, y=w996) -> (x .and. y?=w992:bool)
        n501 = And(x=w993, y=w992) -> (x .and. y?=w991:bool)
        n502 = local write "手动暂停"(w991) -> ()
      }
    }
    n503 = Open/Create/Replace File(file path (use dialog)=path "D:/faster-rcnn.pytorch-pytorch-1.0/data.txt" ("文件路径（使用对话框）")) -> (refnum out=w756:refnum<file>)  [unwired: 5 in, 2 out]
    n504 = case shown="真" "图像检测" {
      tunnel: w769 -> [_ w827]
      tunnel: w756 -> [w823 w826]
      tunnel: [w823 w825] -> w755
      tunnel: w751 -> [_ w824]
      frame False {
      }
      frame True {
        n505 = stacked-sequence {
          tunnel: w827 -> [_ _ _ w863 _ _]
          tunnel: w826 -> [_ _ w835 _ _ _]
          tunnel: [_ _ w834 _ _ _] -> w825
          tunnel: w824 -> [_ _ _ w856 _ _]
          frame #0 {
            n506 = local read "Image"() -> (w829:T4)
            n507 = call-poly "IMAQ Write File 2"("File Path"=path "D:/faster-rcnn.pytorch-pytorch-1.0/temp_img/img.png", "Image"=w829) -> ()  [unwired: 8 in, 2 out]
          }
          frame #1 {
            # "等待rcnn预测"
            n508 = Wait (ms)(milliseconds to wait=u32 1000 ("等待时间（毫秒）")) -> ()  [unwired: 1 out]
          }
          frame #2 {
            w842 = 100 ("y")
            n509 = Set File Position(refnum=w835, from (0:start)=enum16{"start", "end", "current"}."start" ("自（0:起始）")) -> (refnum out=w852:refnum<file>, error out=w854:errorcluster)  [unwired: 2 in]
            n510 = Read from Text File(file (use dialog)=w852, count=1 ("计数"), error in=w854) -> (refnum out=w834:refnum<file>, text=w845:string[], error out=→"错误输出 2":errorcluster)  [unwired: 1 in, 1 out]
            n511 = Index Array(array=w845, index=0 ("索引")) -> (element=w840:string)
            n512 = Match Pattern(string=w840, regular expression="," ("正则表达式")) -> (before substring=w839:string, after substring=w838:string)  [unwired: 1 in, 2 out]
            n513 = Decimal String To Number(string=w839) -> (number=w832:i32)  [unwired: 2 in, 1 out]
            "X 2" <- w832
            n514 = Decimal String To Number(string=w838) -> (number=w846:i32)  [unwired: 2 in, 1 out]
            "Y 2" <- w846
            n515 = Subtract(x=w832, y=w842) -> (x-y=w843:i32)
            n516 = Subtract(x=w846, y=w842) -> (x-y=w849:i32)
            n517 = Add(x=w832, y=w842) -> (x+y=w850:i32)
            n518 = Add(x=w846, y=w842) -> (x+y=w848:i32)
            n519 = To Long Integer(number=w843) -> (32bit integer=w844:i32)
            n520 = To Long Integer(number=w849) -> (32bit integer=w837:i32)
            n521 = To Long Integer(number=w850) -> (32bit integer=w836:i32)
            n522 = To Long Integer(number=w848) -> (32bit integer=w847:i32)
            n523 = Build Array(w844, w837, w836, w847) -> (→"裁剪数组":i32[])
          }
          frame #3 {
            w859 = -1 ("y")
            n524 = local read "Y 2"() -> (w860:i32)
            n525 = local read "X 2"() -> (w857:i32)
            n526 = Equal?(x=w857, y=w859) -> (x = y?=w861:bool)
            n527 = Equal?(x=w860, y=w859) -> (x = y?=w862:bool)
            n528 = Or(x=w861, y=w862) -> (x .or. y?=w858:bool)
            n529 = case shown="真" w858 {
              tunnel: w863 -> [w885 _]
              tunnel: w856 -> [w867 _]
              frame False {
                (unwired) "hello" ("数据输入")
                (unwired) "10.134.224.218" ("名称")
                # "tcp通信"
                # "tcp通信"
                n530 = local read "裁剪数组"() -> (w864:i32[])
                n531 = local read "Image"() -> (w886:T4)
                n532 = call "IMAQ Extract 2"("Optional Rectangle"=w864, "Image Dst"=w885, "Image Src"=w886) -> ("Image Dst Out"=w866:T4)  [unwired: 7 in, 1 out]
                n533 = call "IMAQ Resample"("X Resolution"=128, "Y Resolution"=128, "Image Dst"=w867, "Image Src"=w866) -> ("Image Dst Out"=w865:T4)  [unwired: 6 in, 1 out]
                n534 = call "IMAQ ImageToArray"("Image"=w865) -> ("Image Pixels (U8)"=w881:u8[][])  [unwired: 3 in, 4 out]
                n535 = for {
                  tunnel: w881 -> [w912] mode=indexing
                  tunnel: [w911] -> w883 mode=indexing
                  n536 = for {
                    tunnel: w912 -> [w913] mode=indexing
                    tunnel: [w914] -> w911 mode=indexing
                    n537 = Less?(x=w913, y=u8 10) -> (x < y?=w915:bool)
                    n538 = case shown="假" w915 {
                      tunnel: [w917 w929] -> w914
                      tunnel: w913 -> [w918 w930]
                      frame False {
                        n539 = Less?(x=w918, y=u8 100) -> (x < y?=w919:bool)
                        n540 = case shown="真" w919 {
                          tunnel: w918 -> [w922 w924]
                          tunnel: [w921 w923] -> w917
                          frame False {
                            n541 = Number To Decimal String(number=w922) -> (decimal integer string=w921:string)  [unwired: 1 in]
                          }
                          frame True {
                            n542 = Number To Decimal String(number=w924) -> (decimal integer string=w926:string)  [unwired: 1 in]
                            n543 = Concatenate Strings("0" ("字符串"), w926) -> (w923:string)
                          }
                        }
                      }
                      frame True {
                        n544 = Number To Decimal String(number=w930) -> (decimal integer string=w928:string)  [unwired: 1 in]
                        n545 = Concatenate Strings("00" ("字符串"), w928) -> (w929:string)
                      }
                    }
                  }
                }
                n546 = Add(x="发送次数", y=1.0) -> (x+y=w868:dbl)
                n547 = local write "发送次数"(w868) -> ()
                n548 = Concatenate Strings(w883) -> (w880:string)
                n549 = TCP Open Connection(address="10.134.24.208" ("名称"), remote port or service name=u16 8888 ("远程端口或服务名称")) -> (connection ID=w879:refnum<k5>, error out=w878:errorcluster)  [unwired: 3 in]
                n550 = TCP Write(connection ID=w879, data in=w880, error in (no error)=w878) -> (connection ID out=w876:refnum<k5>, bytes written=→"写入的字节":i32, error out=w877:errorcluster)  [unwired: 1 in]
                n551 = case shown="无错误" w877 {
                  selector: w877 -> [w905 _]
                  tunnel: [w895 errorcluster {"status"=FALSE, "code"=0, "source"=""} ("error IO")] -> w875
                  tunnel: [w897 w909] -> w874
                  tunnel: w876 -> [w894 w909]
                  frame No Error {
                    w891 = 1.5625
                    n552 = TCP Read(connection ID=w894, bytes to read=7 ("读取的字节"), error in (no error)=w905) -> (connection ID out=w897:refnum<k5>, data out=w898:string, error out=w896:errorcluster)  [unwired: 2 in]
                    "数据输出 3" <- w898
                    n553 = case shown="无错误" w896 {
                      selector: w896 -> [w907 _]
                      tunnel: [w907 errorcluster {"status"=FALSE, "code"=0, "source"=""} ("error IO")] -> w895
                      frame No Error {
                      }
                      frame Error {
                      }
                    }
                    n554 = String Subset(string=w898, offset (0)=4 ("偏移量(0)"), length (rest)=3 ("长度（剩余）")) -> (substring=w899:string)
                    n555 = String Subset(string=w898, offset (0)=1 ("偏移量(0)"), length (rest)=3 ("长度（剩余）")) -> (substring=w902:string)
                    n556 = Decimal String To Number(string=w899) -> (number=w888:i32)  [unwired: 2 in, 1 out]
                    n557 = Decimal String To Number(string=w902) -> (number=w887:i32)  [unwired: 2 in, 1 out]
                    n558 = Multiply(x=w888, y=w891) -> (x*y=w892:dbl)
                    n559 = Multiply(x=w887, y=w891) -> (x*y=w893:dbl)
                    n560 = Round To Nearest(number=w892) -> (nearest integer value=→"Y 3":dbl)
                    n561 = Round To Nearest(number=w893) -> (nearest integer value=→"X 3":dbl)
                  }
                  frame Error {
                  }
                }
                "error IO" <- w875
                n562 = TCP Close Connection(connection ID=w874, error in (no error)=w875) -> ()  [unwired: 1 in, 2 out]
              }
              frame True {
              }
            }
          }
          frame #4 {
            w933 = -1 ("y")
            n563 = local read "X 3"() -> (w944:i32)
            n564 = local read "Y 3"() -> (w942:i32)
            n565 = local read "X 2"() -> (w937:i32)
            n566 = local read "Y 2"() -> (w936:i32)
            n567 = Equal?(x=w937, y=w933) -> (x = y?=w935:bool)
            n568 = Equal?(x=w936, y=w933) -> (x = y?=w934:bool)
            n569 = Equal?(x=w944, y=0) -> (x = y?=w940:bool)
            n570 = Equal?(x=w942, y=0) -> (x = y?=w939:bool)
            n571 = Or(x=w935, y=w934) -> (x .or. y?=w932:bool)
            n572 = And(x=w940, y=w939) -> (x .and. y?=w938:bool)
            n573 = Or(x=w938, y=w932) -> (x .or. y?=w931:bool)
            n574 = case shown="假" w931 {
              frame False {
                n575 = flat-sequence {
                  frame #0 {
                    "图像检测到" <- TRUE
                  }
                  frame #1 {
                    n576 = local write "图像检测"(FALSE) -> ()
                  }
                }
                n577 = local read "X 2"() -> (w955:i32)
                n578 = local read "X 3"() -> (w954:i32)
                n579 = local read "Y 2"() -> (w953:i32)
                n580 = local read "Y 3"() -> (w952:i32)
                n581 = Add(x=w955, y=w954) -> (x+y=w949:i32)
                n582 = Add(x=w953, y=w952) -> (x+y=w948:i32)
                n583 = Subtract(x=w949, y=100) -> (x-y=w946:i32)
                n584 = Subtract(x=w948, y=100) -> (x-y=w945:i32)
                n585 = Build Array(w946, w945) -> (w947:i32[])
                n586 = local write "目标坐标"(w947) -> ()
              }
              frame True {
              }
            }
          }
          frame #5 {
            n587 = local write "图像检测"(FALSE) -> ()
          }
        }
      }
    }
    n588 = Close File(refnum=w755) -> ()  [unwired: 1 in, 2 out]
  }
  n589 = call "IMAQ Dispose"("Image"=w142, "error in (no error)"=w141) -> ("error out"=w147:errorcluster)  [unwired: 4 in]
  n590 = call <vilib>:"IMAQdx Close Camera.vi"("error in"=w139, "Session In"=w146) -> ("error out"=w148:errorcluster)  [unwired: 9 in]
  n591 = Release Queue(queue=w136, error in (no error)=w135) -> (error out=w86:errorcluster)  [unwired: 1 in, 2 out]
  n592 = Merge Errors(w147, w148, w86) -> (→"错误输出":errorcluster)
  n593 = Get Date/Time String(date format (0)=enum16{"short", "long", "abbreviated"}."long" ("日期格式(0)"), want seconds? (F)=TRUE ("需要秒？(F)")) -> (date string=w72:string, time string=w57:string)  [unwired: 1 in]
  n594 = String Subset(string=w57, offset (0)=6 ("偏移量(0)")) -> (substring=w55:string)  [unwired: 1 in]
  n595 = String Subset(string=w57, offset (0)=3 ("偏移量(0)"), length (rest)=2 ("长度（剩余）")) -> (substring=w67:string)
  n596 = String Subset(string=w57, length (rest)=2 ("长度（剩余）")) -> (substring=w69:string)  [unwired: 1 in]
  n597 = Concatenate Strings(w69, "时" ("字符串"), w67, "分" ("字符串"), w55, "秒" ("字符串")) -> (w68:string)
  n598 = Concatenate Strings(w72, w68) -> (w51:string)
  n599 = Build Path(base path=path "D:/韩宇/实验/数据" ("文件路径（使用对话框）"), name or relative path=w51) -> (appended path=w65:path)
  n600 = Create Folder(path (use dialog)=w65) -> (created path=w60:path)  [unwired: 2 in, 2 out]
  n601 = Build Path(base path=w60, name or relative path="data.txt" ("字符串")) -> (appended path=w62:path)
  n602 = Open/Create/Replace File(file path (use dialog)=w62, operation (0:open)=T8."open or create" ("操作(0:open)")) -> (refnum out=w61:refnum<file>)  [unwired: 4 in, 2 out]
  n603 = while {
    tunnel: w39 -> [w1077]
    tunnel: w40 -> [w1091]
    tunnel: w41 -> [w1090]
    tunnel: w61 -> [w1085]
    tunnel: w60 -> [w1084]
    tunnel: [w1076] -> w59
    tunnel: w38 -> [w1082]
    tunnel: [w1078] -> w35
    tunnel: w33 -> [w1061]
    tunnel: [w1075] -> w34
    tunnel: w33 -> [w1064]
    tunnel: w27 -> [w1069]
    tunnel: w26 -> [w1068]
    tunnel: [w1069] -> w25
    tunnel: [w1068] -> w24
    i -> [w1083]
    stop <- w1092 stop-if-true
    # "Mp285A控制循环"
    n604 = Dequeue Element(queue=w1090, timeout in ms (-1)=1 ("超时毫秒(-1)"), error in (no error)=w1091) -> (error out=w1093:errorcluster)  [unwired: 3 out]
    n605 = Unbundle By Name(w1093) -> ("status"=w1092:bool)
    n606 = event shown="[4] \"针尖粗对焦\": 值改变" {
      selector: _ -> [_ _ _ _ _ _]
      dyn-events: _ -> [_ _ _ _ _ _]
      timeout: 1 -> [_ _ _ _ _ _]
      event "自动接触": Value Change {
        # "事件结构有问题"
        n607 = event-data() -> ()  [unwired: 1 in, 6 out]
        n608 = local read "Resistance(MΩ)"() -> (w1106:dbl)
        n609 = Greater?(x=w1106, y=15.0) -> (0:w1103:bool)
        n610 = Less?(x=w1106, y=3.0) -> (x < y?=w1102:bool)
        n611 = Or(x=w1103, y=w1102) -> (x .or. y?=w1101:bool)
        n612 = local write "校准的入液阻值"(w1106) -> ()
        n613 = case shown="真" w1101 {
          frame False {
          }
          frame True {
            n614 = local write "自动接触"(FALSE) -> ()
            n615 = One Button Dialog(message="针尖异常" ("消息")) -> ()  [unwired: 1 in, 1 out]
          }
        }
        "自动接触初始" <- 0
        "针下降次数" <- 0 ("针下降次数")
      }
      event "傅里叶": Value Change {
        w1111 = u16 0 items=["傅里叶初始", "傅里叶循环", "傅里叶暂停", "傅里叶结束"] ("傅里叶状态机")
        n616 = event-data() -> ()  [unwired: 1 in, 6 out]
        n617 = local write "傅里叶状态机"(w1111) -> ()
      }
      event Timeout {
        n618 = event-data() -> ()  [unwired: 1 in, 3 out]
      }
      event "自动扫描": Value Change {
        w1112 = u16 0 items=["自动扫描初始", "自动扫描循环", "自动扫描结束"] ("自动扫描状态机")
        n619 = event-data() -> ()  [unwired: 1 in, 6 out]
        n620 = local write "自动扫描状态机"(w1112) -> ()
      }
      event "针尖粗对焦": Value Change {
        w1113 = u16 0 items=["自动对焦初始", "自动对焦循环", "自动对焦结束"] ("自动对焦状态机")
        n621 = event-data() -> ()  [unwired: 1 in, 6 out]
        n622 = local write "自动对焦状态机"(w1113) -> ()
      }
      event "升Z轴找针": Value Change {
        w1114 = u16 0 items=["升Z轴找针初始", "升Z轴找针循环", "升Z轴找针结束"] ("升Z轴找针状态机")
        n623 = event-data() -> ()  [unwired: 1 in, 6 out]
        n624 = local write "升Z轴找针状态机"(w1114) -> ()
        n625 = local write "没匹配到？"(TRUE) -> ()
      }
    }
    n626 = case shown="真" "移至工作位置" {
      tunnel: w1082 -> [w1354 w1363]
      tunnel: w1077 -> [w1355 w1360]
      tunnel: [w1355 w1357] -> w1079
      tunnel: [w1354 w1356] -> w1078
      frame False {
      }
      frame True {
        n627 = flat-sequence {
          tunnel: w1363 -> [w1366]
          tunnel: [w1364] -> w1362
          tunnel: w1362 -> [w1373]
          tunnel: [w1373] -> w1361
          tunnel: w1361 -> [w1383]
          tunnel: w1360 -> [w1382]
          tunnel: [w1383] -> w1359
          tunnel: [w1378] -> w1358
          tunnel: [w1385] -> w1357
          tunnel: [w1386] -> w1356
          tunnel: w1359 -> [w1386]
          tunnel: w1358 -> [w1385]
          frame #0 {
            n628 = call "285_GetPos.vi"("VISA资源名称"=w1366) -> ("Y"=→"Y":dbl, "X"=→"X":dbl, "VISA资源名称输出"=w1364:refnum<visa-resource-name>)  [unwired: 5 in, 3 out]
          }
          frame #1 {
            n629 = local read "Z轴坐标"() -> (w1369:string)
            n630 = Decimal String To Number(string=w1369) -> (number=w1368:i32)  [unwired: 2 in, 1 out]
            n631 = To Double Precision Float(number=w1368) -> (double precision float=w1370:dbl)
            n632 = Divide(x=w1370, y=10.0) -> (x/y=→"Z":dbl)
          }
          frame #2 {
            # "等待针尖到达延时"
            # "标定"
            n633 = local read "Z"() -> (w1379:dbl)
            n634 = local read "Y"() -> (w1380:dbl)
            n635 = local read "X"() -> (w1381:dbl)
            n636 = Add(x=w1379, y="z输入") -> ()  [unwired: 1 out]
            n637 = Add(x=w1380, y="y输入") -> ()  [unwired: 1 out]
            n638 = Add(x=w1381, y="x输入") -> ()  [unwired: 1 out]
            n639 = call "285_Move.vi"("VISA resource name out"=w1382, "Abso_Z"="z输入", "Abso_Y"="y输入", "Abso_X"="x输入") -> ("VISA resource name out 2"=w1378:refnum<visa-resource-name>)  [unwired: 4 in, 3 out]
            n640 = Wait (ms)(milliseconds to wait=u32 5000 ("等待时间（毫秒）")) -> ()  [unwired: 1 out]
          }
          frame #3 {
            n641 = disable-structure shown="启用" {
              frame Disabled {
              }
              frame Enabled {
                n642 = local write "自动扫描"(TRUE ("自动扫描")) -> ()
              }
            }
            n643 = local write "移至工作位置"(FALSE) -> ()
          }
        }
      }
    }
    n644 = flat-sequence {
      tunnel: w1077 -> [w1478]
      tunnel: [w1475] -> w1066
      tunnel: [w1519] -> w1089
      tunnel: w1066 -> [w1516]
      frame #0 {
        n645 = local read "Right"() -> (w1476:dbl)
        n646 = case shown="真" "针尖粗对焦" {
          tunnel: w1478 -> [w1479 w1482]
          tunnel: w1476 -> [_ w1483]
          tunnel: [w1479 w1481] -> w1475
          frame False {
          }
          frame True {
            n647 = case shown="1" "自动对焦状态机" {
              tunnel: w1483 -> [w1494 w1497]
              frame 0, Default {
                w1495 = u16 1 items=["自动对焦初始", "自动对焦循环", "自动对焦结束"] ("自动对焦状态机")
                n648 = local write "自动对焦状态机"(w1495) -> ()
                "right_old" <- w1494
                "调焦值上升过？" <- FALSE
                "对焦变量" <- 1
              }
              frame 1 {
                n649 = local read "right_old"() -> (w1505:dbl)
                n650 = local read "right_old"() -> (w1500:dbl)
                n651 = Add(x=w1505, y=40.0) -> (x+y=w1503:dbl)
                n652 = Subtract(x=w1500, y=40.0) -> (x-y=w1499:dbl)
                n653 = Less?(x=w1497, y=w1499) -> (x < y?=w1498:bool)
                n654 = Greater?(x=w1497, y=w1503) -> (0:w1502:bool)
                n655 = case shown="真" w1502 {
                  tunnel: w1497 -> [_ w1515]
                  frame False {
                  }
                  frame True {
                    n656 = local write "调焦值上升过？"(TRUE ("调焦值上升过？")) -> ()
                    n657 = local write "right_old"(w1515) -> ()
                  }
                }
                n658 = case shown="真" w1498 {
                  tunnel: w1497 -> [_ w1507]
                  frame False {
                  }
                  frame True {
                    n659 = local write "right_old"(w1507) -> ()
                    n660 = local read "调焦值上升过？"() -> (w1506:bool)
                    n661 = case shown="真" w1506 {
                      frame False {
                        n662 = local read "对焦变量"() -> (w1510:dbl)
                        n663 = Multiply(x=w1510, y=-1.0) -> (x*y=w1509:dbl)
                        n664 = local write "对焦变量"(w1509) -> ()
                      }
                      frame True {
                        w1511 = u16 0 items=["自动对焦初始", "自动对焦循环", "自动对焦结束"] ("自动对焦状态机")
                        n665 = local write "针尖粗对焦"(FALSE ("针尖粗对焦")) -> ()
                        n666 = local write "针尖细对焦"(TRUE ("针尖细对焦")) -> ()
                        n667 = local write "自动对焦状态机"(w1511) -> ()
                      }
                    }
                  }
                }
              }
            }
            n668 = local read "针尖粗对焦"() -> (w1480:bool)
            n669 = case shown="假" w1480 {
              tunnel: w1482 -> [w1485 w1488]
              tunnel: [w1485 w1487] -> w1481
              frame False {
              }
              frame True {
                n670 = local read "对焦变量"() -> (w1486:dbl)
                n671 = Multiply(x=5.0 ("Z 2"), y=w1486) -> (x*y=w1492:dbl)
                n672 = call "285_RelMove.vi"("VISA资源名称"=w1488, "Z 2"=w1492, "Y 2"=0.0, "X 2"=0.0) -> ("VISA resource name out 2"=w1487:refnum<visa-resource-name>)  [unwired: 2 in, 5 out]
              }
            }
          }
        }
      }
      frame #1 {
        n673 = case shown="真" "针尖细对焦" {
          tunnel: [w1520 w1521] -> w1519
          tunnel: w1516 -> [w1520 w1522]
          frame False {
          }
          frame True {
            n674 = local read "没匹配到？"() -> (w1523:bool)
            n675 = case shown="假" w1523 {
              tunnel: [w1524 w1533] -> w1521
              tunnel: w1522 -> [w1524 w1527]
              frame False {
                n676 = disable-structure shown="启用" {
                  frame Disabled {
                  }
                  frame Enabled {
                    n677 = local write "针尖移动"(TRUE ("针尖自动移动")) -> ()
                  }
                }
                n678 = local write "针尖细对焦"(FALSE ("针尖细对焦")) -> ()
              }
              frame True {
                n679 = local read "对焦变量"() -> (w1530:dbl)
                n680 = Multiply(x=-1.0, y=w1530) -> (x*y=w1528:dbl)
                n681 = call "285_RelMove.vi"("VISA资源名称"=w1527, "Z 2"=w1528, "Y 2"=0.0, "X 2"=0.0) -> ("VISA resource name out 2"=w1533:refnum<visa-resource-name>)  [unwired: 2 in, 5 out]
              }
            }
          }
        }
        n682 = Wait (ms)(milliseconds to wait=u32 200 ("等待时间（毫秒）")) -> ()  [unwired: 1 out]
      }
    }
    n683 = case shown="真" "自动扫描" {
      tunnel: w1079 -> [_ w1313]
      frame False {
      }
      frame True {
        n684 = case shown="2" "自动扫描状态机" {
          tunnel: w1313 -> [w1314 w1323 _]
          frame 0, Default {
            # "初始状态"
            n685 = flat-sequence {
              tunnel: w1314 -> [w1316]
              frame #0 {
                n686 = call "285_RelMove.vi"("VISA资源名称"=w1316, "Z 2"=0.0, "Y 2"=300.0 ("X 2"), "X 2"=0.0 ("Y 2")) -> ()  [unwired: 2 in, 6 out]
                "扫描变量" <- -1.0 ("扫描变量")
              }
              frame #1 {
                n687 = local write "自动扫描状态机"(u16 1) -> ()
                n688 = Wait (ms)(milliseconds to wait=u32 1000 ("等待时间（毫秒）")) -> ()  [unwired: 1 out]
              }
              frame #2 {
              }
            }
          }
          frame 1 {
            n689 = case shown="假" "手动暂停" {
              tunnel: w1323 -> [w1325 _]
              frame False {
                n690 = flat-sequence {
                  tunnel: [w1327] -> w1324
                  tunnel: w1325 -> [w1328]
                  tunnel: w1324 -> [w1340]
                  tunnel: [w1339] -> _
                  frame #0 {
                    n691 = for {
                      N: 30 -> [_]
                      shift-right: [w1336] -> w1327
                      shift-left: w1328 -> [w1337]
                      stop <- w1329 stop-if-true
                      n692 = local read "手动暂停"() -> (w1329:bool)
                      n693 = local read "扫描变量"() -> (w1333:dbl)
                      n694 = Multiply(x=20.0 ("X 2"), y=w1333) -> (x*y=w1331:dbl)
                      n695 = Wait (ms)(milliseconds to wait=u32 50 ("等待时间（毫秒）")) -> ()  [unwired: 1 out]
                      n696 = call "285_RelMove.vi"("VISA资源名称"=w1337, "Z 2"=0.0, "Y 2"=w1331, "X 2"=0.0 ("Y 2")) -> ("VISA resource name out 2"=w1336:refnum<visa-resource-name>)  [unwired: 2 in, 5 out]
                    }
                  }
                  frame #1 {
                    n697 = local read "手动暂停"() -> (w1338:bool)
                    n698 = case shown="假" w1338 {
                      tunnel: w1340 -> [w1348 w1349]
                      tunnel: [w1344 w1349] -> w1339
                      frame False {
                        n699 = call "285_RelMove.vi"("VISA资源名称"=w1348, "Z 2"=0.0, "Y 2"=0.0 ("X 2"), "X 2"=-50.0 ("Y 2")) -> ("VISA resource name out 2"=w1344:refnum<visa-resource-name>)  [unwired: 2 in, 5 out]
                        n700 = local read "扫描变量"() -> (w1343:dbl)
                        n701 = Multiply(x=w1343, y=-1.0) -> (x*y=w1341:dbl)
                        n702 = local write "扫描变量"(w1341) -> ()
                      }
                      frame True {
                      }
                    }
                  }
                }
              }
              frame True {
                n703 = flat-sequence {
                  frame #0 {
                    n704 = local write "自动扫描状态机"(2) -> ()
                  }
                  frame #1 {
                  }
                }
              }
            }
          }
          frame 2 {
            n705 = flat-sequence {
              frame #0 {
                n706 = local write "自动扫描状态机"(0) -> ()
              }
              frame #1 {
                w1352 = FALSE
                n707 = disable-structure shown="启用" {
                  frame Disabled {
                  }
                  frame Enabled {
                    n708 = local write "针尖粗对焦"(TRUE ("针尖粗对焦")) -> ()
                  }
                }
                n709 = local write "自动扫描"(w1352) -> ()
                n710 = local write "手动暂停"(w1352) -> ()
              }
            }
          }
        }
      }
    }
    n711 = case shown="真" "手动换物镜" {
      tunnel: w1079 -> [_ w1303]
      tunnel: w1061 -> [_ w1302]
      frame False {
      }
      frame True {
        n712 = flat-sequence {
          tunnel: w1303 -> [w1311]
          tunnel: w1302 -> [_]
          frame #0 {
            n713 = One Button Dialog(message="针尖已移动到视野中间位置，\n请手动更换40倍显微镜！" ("消息")) -> ()  [unwired: 1 in, 1 out]
          }
          frame #1 {
            w1305 = u16 0 items=["傅里叶初始", "傅里叶循环", "傅里叶暂停", "傅里叶结束"] ("傅里叶状态机")
            n714 = call "285_RelMove.vi"("VISA资源名称"=w1311, "Z 2"=0.0, "Y 2"=0.0, "X 2"=0.0) -> ()  [unwired: 2 in, 6 out]
            n715 = local write "傅里叶状态机"(w1305) -> ()
            n716 = local write "手动换物镜"(FALSE) -> ()
            n717 = local write "傅里叶"(TRUE) -> ()
          }
        }
      }
    }
    n718 = disable-structure shown="禁用" {
      frame Disabled {
      }
      frame Enabled {
      }
    }
    n719 = case shown="假" "针尖移动 2" {
      tunnel: [sgl[] [1536.0, 1024.0] ("针尖坐标") w1119] -> w1088
      tunnel: [100.0 ("y") 10.0 ("y")] -> w1060
      frame False {
        # "图像中间坐标"
      }
      frame True {
        n720 = local read "目标坐标"() -> (w1119:i32[])
      }
    }
    n721 = local read "针尖坐标"() -> (w1072:sgl[])
    n722 = Or(x="针尖移动", y="针尖移动 2") -> (x .or. y?=w1074:bool)
    n723 = case shown="真" "傅里叶" {
      tunnel: w1061 -> [_ w1191]
      tunnel: w1069 -> [_ w1190]
      tunnel: w1068 -> [_ w1189]
      frame False {
      }
      frame True {
        n724 = case shown="2" "傅里叶状态机" {
          tunnel: w1191 -> [w1193 w1224 _ _]
          tunnel: w1190 -> [_ w1219 _ _]
          tunnel: w1189 -> [_ w1218 _ _]
          frame 0, Default {
            n725 = flat-sequence {
              tunnel: w1193 -> [w1199]
              frame #0 {
                n726 = call "SetZ_step.vi"("step"=2000, "VISA资源名称"=w1199) -> ("VISA资源名称输出"=w1198:refnum<visa-resource-name>)  [unwired: 8 in, 1 out]
                n727 = Concatenate Strings("D" ("写入缓冲区"), "\r") -> (w1208:string)
                n728 = VISA Write ("VISA写入")(VISA resource name=w1198, write buffer=w1208) -> (VISA resource name out=w1205:refnum<visa-resource-name>, error out=w1204:errorcluster)  [unwired: 1 in, 1 out]
                n729 = property class="Instr"(reference=w1205, error in=w1204) -> (reference out=w1207:refnum<visa-resource-name>, error out=w1203:errorcluster, "Serial Settings:Number of Bytes at Serial Port"=w1206:u32)
                n730 = VISA Read(VISA resource name=w1207, byte count=w1206, error in (no error)=w1203) -> (VISA resource name out=w1197:refnum<visa-resource-name>, error out=w1196:errorcluster)  [unwired: 2 out]
                n731 = call "SetZ_step.vi"("错误输入（无错误）"=w1196, "step"=20, "VISA资源名称"=w1197) -> ()  [unwired: 7 in, 2 out]
                n732 = Wait (ms)(milliseconds to wait=u32 2000 ("等待时间（毫秒）")) -> ()  [unwired: 1 out]
              }
              frame #1 {
                w1214 = FALSE
                n733 = Build Array(w1214, w1214) -> (→"傅里叶数组":bool[])
                n734 = local write "没有细胞"(FALSE ("没有细胞")) -> ()
                n735 = local write "目标坐标"(i32[] [0, 0] ("目标坐标")) -> ()
                "物镜下降次数" <- 0
                "傅里叶最大值" <- 0.0
                "已发送图像" <- FALSE ("已发送图像")
              }
              frame #2 {
                w1216 = u16 1 items=["傅里叶初始", "傅里叶循环", "傅里叶暂停", "傅里叶结束"] ("傅里叶状态机")
                n736 = local write "傅里叶状态机"(w1216) -> ()
              }
            }
          }
          frame 1 {
            n737 = flat-sequence {
              tunnel: w1224 -> [w1227]
              tunnel: [w1226] -> w1223
              tunnel: w1223 -> [w1240]
              tunnel: [w1239] -> w1217
              tunnel: [w1245] -> w1222
              tunnel: w1219 -> [w1266]
              tunnel: w1218 -> [w1267]
              tunnel: w1217 -> [w1248]
              tunnel: w1222 -> [w1272]
              tunnel: [w1274] -> w1221
              tunnel: [w1273] -> w1220
              tunnel: w1221 -> [w1283]
              tunnel: w1220 -> [w1282]
              frame #0 {
                n738 = local read "已发送图像"() -> (w1225:bool)
                n739 = case shown="假" w1225 {
                  frame False {
                    # "记录下降多少"
                    n740 = local read "物镜下降次数"() -> (w1238:i32)
                    n741 = Add(x=w1238, y=1) -> (x+y=w1237:i32)
                    n742 = local write "物镜下降次数"(w1237) -> ()
                  }
                  frame True {
                  }
                }
                n743 = Concatenate Strings("D" ("写入缓冲区"), "\r") -> (w1235:string)
                n744 = VISA Write ("VISA写入")(VISA resource name=w1227, write buffer=w1235) -> (VISA resource name out=w1230:refnum<visa-resource-name>, error out=w1232:errorcluster)  [unwired: 1 in, 1 out]
                n745 = property class="Instr"(reference=w1230, error in=w1232) -> (reference out=w1233:refnum<visa-resource-name>, error out=w1234:errorcluster, "Serial Settings:Number of Bytes at Serial Port"=w1231:u32)
                n746 = VISA Read(VISA resource name=w1233, byte count=w1231, error in (no error)=w1234) -> (VISA resource name out=w1226:refnum<visa-resource-name>)  [unwired: 3 out]
              }
              frame #1 {
                n747 = VISA Flush I/O Buffer(VISA resource name=w1240) -> (VISA resource name out=w1239:refnum<visa-resource-name>)  [unwired: 2 in, 1 out]
                n748 = Wait (ms)(milliseconds to wait=u32 100 ("等待时间（毫秒）")) -> ()  [unwired: 1 out]
              }
              frame #2 {
                n749 = local read "Image"() -> (w1251:T4)
                n750 = call "IMAQ ImageToArray"("Image"=w1251) -> ("error out"=w1258:errorcluster, "Image Pixels (U8)"=w1250:u8[][])  [unwired: 3 in, 3 out]
                n751 = call "IMAQ ArrayToComplexPlane"("Plane"=enum32{"Real", "Imaginary"}."Real", "Image"=w1267, "Image Pixels (float)"=w1250, "error in (no error)"=w1258) -> ("Image Out"=w1256:T4)  [unwired: 1 in, 1 out]
                n752 = call "IMAQ FFT"("Image Dst"=w1266, "Image Src"=w1256) -> ("error out"=w1255:errorcluster, "Image Dst Out"=w1254:T4)  [unwired: 2 in]
                n753 = local read "傅里叶最大值"() -> (w1249:dbl)
                n754 = call "IMAQ ComplexPlaneToArray"("error in (no error)"=w1255, "Plane"=T12."Magnitude", "Image"=w1254) -> ("Image Pixels (float)"=w1252:sgl[][])  [unwired: 2 in, 1 out]
                n755 = Add Array Elements(numeric array=w1252) -> (sum=w1247:sgl)
                "傅里叶求和" <- w1247
                n756 = Greater?(x=w1249, y=w1247) -> (0:w1261:bool)
                n757 = Select(t=w1249, s=w1261, f=w1247) -> (s? t:f=w1242:dbl)
                n758 = Less?(x=w1247, y=w1242) -> (x < y?=w1246:bool)
                n759 = local write "傅里叶最大值"(w1242) -> ()
                n760 = Multiply(x=w1242, y=0.96) -> (x*y=w1262:dbl)
                n761 = Multiply(x=w1242, y=0.998) -> (x*y=w1263:dbl)
                n762 = Less?(x=w1262, y=w1247) -> (x < y?=w1264:bool)
                n763 = Less?(x=w1247, y=w1263) -> (x < y?=w1265:bool)
                n764 = And(x=w1264, y=w1265) -> (x .and. y?=w1245:bool)
                n765 = Not(x=w1245) -> (.not. x?=w1244:bool)
                n766 = And(x=w1244, y=w1246) -> (x .and. y?=w1243:bool)
                n767 = case shown="真" w1243 {
                  tunnel: w1248 -> [_ w1268]
                  frame False {
                  }
                  frame True {
                    n768 = call "SetZ_step.vi"("step"=20, "VISA资源名称"=w1268) -> ()  [unwired: 8 in, 2 out]
                  }
                }
              }
              frame #3 {
                n769 = local read "傅里叶数组"() -> (w1277:bool[])
                n770 = local read "已发送图像"() -> (w1270:bool)
                n771 = Insert Into Array(array=w1277, index=0 ("索引"), new element=w1272) -> (w1276:bool[])
                n772 = And Array Elements(Boolean array=w1277) -> (logical AND=w1281:bool)
                n773 = Or Array Elements(Boolean array=w1277) -> (logical OR=w1280:bool)
                n774 = And(x=w1272, y=w1281) -> (x .and. y?=w1274:bool)
                n775 = Not Or(1:w1280, 2:w1272) -> (0:w1279:bool)
                n776 = Delete From Array(array=w1276) -> (array with subset deleted=w1275:bool[])  [unwired: 2 in, 1 out]
                n777 = Or(x=w1274, y=w1270) -> (x .or. y?=w1271:bool)
                n778 = And(x=w1270, y=w1279) -> (x .and. y?=w1273:bool)
                n779 = local write "已发送图像"(w1271) -> ()
                n780 = local write "傅里叶数组"(w1275) -> ()
              }
              frame #4 {
                n781 = case shown="真" w1282 {
                  frame False {
                  }
                  frame True {
                    n782 = flat-sequence {
                      frame #0 {
                        n783 = One Button Dialog(message="没有细胞！！" ("消息")) -> ()  [unwired: 1 in, 1 out]
                        n784 = local write "没有细胞"(TRUE) -> ()
                      }
                      frame #1 {
                        w1286 = u16 0 items=["傅里叶初始", "傅里叶循环", "傅里叶暂停", "傅里叶结束"] ("傅里叶状态机")
                        n785 = local write "傅里叶状态机"(w1286) -> ()
                        n786 = local write "傅里叶"(FALSE ("傅里叶")) -> ()
                      }
                    }
                  }
                }
                n787 = case shown="真" w1283 {
                  frame False {
                  }
                  frame True {
                    w1289 = u16 2 items=["傅里叶初始", "傅里叶循环", "傅里叶暂停", "傅里叶结束"] ("傅里叶状态机")
                    n788 = local write "傅里叶状态机"(w1289) -> ()
                    n789 = local write "图像检测"(TRUE ("升Z轴找针")) -> ()
                    n790 = local write "图像检测到"(FALSE) -> ()
                  }
                }
              }
            }
          }
          frame 2 {
            n791 = local read "图像检测到"() -> (w1293:bool)
            n792 = local read "图像检测"() -> (w1291:bool)
            n793 = Not(x=w1291) -> (.not. x?=w1295:bool)
            n794 = And(x=w1293, y=w1295) -> (x .and. y?=w1294:bool)
            n795 = Or(x=w1291, y=w1293) -> (x .or. y?=w1292:bool)
            n796 = case shown="真" w1294 {
              frame False {
              }
              frame True {
                w1297 = u16 3 items=["傅里叶初始", "傅里叶循环", "傅里叶暂停", "傅里叶结束"] ("傅里叶状态机")
                n797 = local write "傅里叶状态机"(w1297) -> ()
              }
            }
            n798 = case shown="假" w1292 {
              frame False {
                w1296 = u16 1 items=["傅里叶初始", "傅里叶循环", "傅里叶暂停", "傅里叶结束"] ("傅里叶状态机")
                n799 = local write "傅里叶状态机"(w1296) -> ()
              }
              frame True {
              }
            }
          }
          frame 3 {
            n800 = flat-sequence {
              frame #0 {
                w1299 = u16 0 items=["傅里叶初始", "傅里叶循环", "傅里叶暂停", "傅里叶结束"] ("傅里叶状态机")
                n801 = local write "傅里叶"(FALSE ("傅里叶")) -> ()
                n802 = local write "傅里叶状态机"(w1299) -> ()
              }
              frame #1 {
                w1300 = u16 0 items=["升Z轴找针初始", "升Z轴找针循环", "升Z轴找针结束"] ("升Z轴找针状态机")
                n803 = local write "升Z轴找针状态机"(w1300) -> ()
                n804 = local write "升Z轴找针"(TRUE ("升Z轴找针")) -> ()
              }
            }
          }
        }
      }
    }
    n805 = case shown="真" w1074 {
      tunnel: w1089 -> [w1425 w1449]
      tunnel: [w1425 w1436] -> w1063
      tunnel: w1088 -> [_ w1438]
      tunnel: w1072 -> [_ w1431]
      tunnel: w1060 -> [_ w1426]
      frame False {
      }
      frame True {
        # "模板针尖偏移量"
        # "PID控制针尖移动"
        # "可以直接用pid模块"
        n806 = Index Array(array=w1431, index=1 ("索引")) -> (element=w1428:sgl)
        n807 = Index Array(array=w1431, index=0 ("索引")) -> (element=w1427:sgl)
        n808 = Index Array(array=w1438, index=1 ("索引")) -> (element=w1447:sgl)
        n809 = Index Array(array=w1438, index=0 ("索引")) -> (element=w1448:sgl)
        n810 = Subtract(x=w1447, y=w1428) -> (x-y=w1443:sgl)
        n811 = Bundle("x"=w1428, "x"=w1447) -> ()  [unwired: 1 in, 1 out]
        n812 = Add(x=sgl 0.0 ("y"), y=w1427) -> (x+y=w1432:sgl)
        n813 = Subtract(x=w1448, y=w1432) -> (x-y=w1444:sgl)
        n814 = call-poly <vilib>:"PID.vi"("PID gains"="PID gains", "process variable"=w1432, "setpoint"=w1448) -> ("output"=w1434:dbl)  [unwired: 7 in, 1 out]
        n815 = call-poly <vilib>:"PID.vi"("PID gains"="PID gains 2", "process variable"=w1428, "setpoint"=w1447) -> ("output"=w1435:dbl)  [unwired: 7 in, 1 out]
        n816 = Bundle("x"=w1427, "x"=w1448) -> ()  [unwired: 1 in, 1 out]
        n817 = Square(x=w1444) -> (x^2=w1442:sgl)
        n818 = Square(x=w1443) -> (x^2=w1441:sgl)
        n819 = Add(x=w1442, y=w1441) -> (x+y=w1437:sgl)
        "x+y" <- w1437
        n820 = Greater?(x=w1437, y=w1426) -> (0:w1450:bool)
        n821 = case shown="假" w1450 {
          tunnel: w1449 -> [w1452 w1461]
          tunnel: [w1452 w1460] -> w1436
          tunnel: w1434 -> [_ w1459]
          tunnel: w1435 -> [_ w1458]
          frame False {
            n822 = local read "针尖移动"() -> (w1451:bool)
            n823 = case shown="假" w1451 {
              frame False {
                n824 = disable-structure shown="启用" {
                  frame Disabled {
                  }
                  frame Enabled {
                    n825 = local write "自动接触"(TRUE ("自动接触")) -> ()
                  }
                }
                n826 = local write "针尖移动 2"(FALSE ("针尖自动移动 2")) -> ()
                n827 = local write "自动接触初始"(0 ("自动接触初始")) -> ()
              }
              frame True {
                n828 = local write "手动换物镜"(TRUE ("手动换物镜")) -> ()
                n829 = local write "针尖移动"(FALSE ("针尖自动移动")) -> ()
              }
            }
          }
          frame True {
            # "阈值范围需要调整，太大针尖检测不出来，太小程序会出现bug'"
            n830 = flat-sequence {
              tunnel: w1461 -> [w1468]
              tunnel: [w1467] -> w1460
              tunnel: w1459 -> [w1463]
              tunnel: w1458 -> [w1462]
              frame #0 {
                # "小距离285不动了？？？"
                # "x位置p负号原因是设备转换后的"
                n831 = To Byte Integer(number=w1462) -> (8bit integer=w1466:i8)
                n832 = To Byte Integer(number=w1463) -> (8bit integer=w1465:i8)
                n833 = In Range and Coerce(upper limit=2.0 ("上限"), x=w1466, lower limit=-2.0 ("上限")) -> (coerced(x)=w1471:dbl)  [unwired: 1 out]
                "已强制转换(y)" <- w1471
                n834 = In Range and Coerce(upper limit=2.0 ("上限"), x=w1465, lower limit=-2.0 ("上限")) -> (coerced(x)=w1464:dbl)  [unwired: 1 out]
                "已强制转换(x)" <- w1464
                n835 = call "285_RelMove.vi"("VISA资源名称"=w1468, "Z 2"=0.0 ("Z"), "Y 2"=w1471, "X 2"=w1464) -> ("VISA resource name out 2"=w1467:refnum<visa-resource-name>)  [unwired: 2 in, 5 out]
              }
            }
          }
        }
      }
    }
    n836 = case shown="真" "自动接触" {
      tunnel: w1063 -> [w1534 w1549]
      tunnel: [w1534 w1545] -> w1087
      tunnel: w1064 -> [_ w1536]
      frame False {
      }
      frame True {
        # "阈值"
        n837 = local read "校准的入液阻值"() -> (w1544:dbl)
        n838 = local read "阻值数组"() -> (w1555:dbl[])
        n839 = local read "自动接触初始"() -> (w1537:i32)
        n840 = Index Array(array=w1555, index=0 ("索引")) -> (element=w1548:dbl)
        n841 = Index Array(array=w1555, index=1 ("索引")) -> (element=w1553:dbl)
        n842 = Index Array(array=w1555, index=2 ("索引")) -> (element=w1552:dbl)
        n843 = Multiply(x=1.1, y=w1544) -> (x*y=w1542:dbl)
        n844 = Greater Or Equal?(x=w1548, y=w1553) -> (x >= y?=w1551:bool)
        n845 = Greater Or Equal?(x=w1553, y=w1552) -> (x >= y?=w1550:bool)
        n846 = Greater?(x=w1548, y=w1542) -> (0:w1547:bool)
        n847 = And(x=w1551, y=w1550) -> (x .and. y?=w1546:bool)
        n848 = And(x=w1547, y=w1546) -> (x .and. y?=w1538:bool)
        n849 = Boolean To (0,1)(Boolean=w1538) -> (0, 1=w1539:i16)
        n850 = Multiply(x=i16 10, y=w1539) -> (x*y=w1540:i16)
        n851 = Add(x=w1540, y=w1537) -> (x+y=w1535:i32)
        "自动接触状态" <- w1535
        n852 = case shown="0, 1, 默认" w1535 {
          tunnel: w1549 -> [w1559 w1604 w1653]
          tunnel: [w1558 w1605 w1653] -> w1545
          tunnel: w1536 -> [_ w1594 _]
          tunnel: w1535 -> [_ w1593 _]
          frame 10 {
            n853 = flat-sequence {
              tunnel: w1559 -> [w1565]
              tunnel: [w1564] -> w1558
              frame #0 {
                # "向下运动"
                n854 = local read "下降/向右"() -> (w1563:bool)
                n855 = local read "针下降次数"() -> (w1562:i32)
                n856 = case shown="真" w1563 {
                  tunnel: [-15.0 ("y") 0.0 ("X 2")] -> w1568
                  tunnel: [0.0 ("X 2") -15.0] -> w1567
                  tunnel: [0.0 ("Y 2") 0.0 ("Y 2")] -> w1566
                  frame False {
                  }
                  frame True {
                  }
                }
                n857 = Subtract(x=w1562, y=15) -> (x-y=w1561:i32)
                n858 = local write "针下降次数"(w1561) -> ()
                n859 = call "285_RelMove.vi"("VISA资源名称"=w1565, "Z 2"=w1568, "Y 2"=w1566, "X 2"=w1567) -> ("VISA resource name out 2"=w1564:refnum<visa-resource-name>)  [unwired: 2 in, 5 out]
              }
              frame #1 {
                n860 = Wait (ms)(milliseconds to wait=u32 3000 ("等待时间（毫秒）")) -> ()  [unwired: 1 out]
              }
              frame #2 {
                # "阈值"
                n861 = local read "校准的入液阻值"() -> (w1588:dbl)
                n862 = local read "阻值数组"() -> (w1586:dbl[])
                n863 = Index Array(array=w1586, index=0 ("索引")) -> (element=w1583:dbl)
                n864 = Index Array(array=w1586, index=1 ("索引")) -> (element=w1582:dbl)
                n865 = Index Array(array=w1586, index=2 ("索引")) -> (element=w1580:dbl)
                n866 = Multiply(x=1.08, y=w1588) -> (x*y=w1581:dbl)
                n867 = Greater?(x=w1581, y=w1582) -> (0:w1579:bool)
                n868 = Greater?(x=w1581, y=w1583) -> (0:w1578:bool)
                n869 = Greater?(x=w1581, y=w1580) -> (0:w1577:bool)
                n870 = Compound Arithmetic op=AND ("复合运算")(w1578, w1579, w1577) -> (w1576:bool)
                n871 = case shown="真" w1576 {
                  frame False {
                    n872 = local write "自动接触"(FALSE ("自动接触")) -> ()
                    n873 = One Button Dialog(message="堵针" ("消息")) -> ()  [unwired: 1 in, 1 out]
                  }
                  frame True {
                    n874 = local write "自动接触初始"(1) -> ()
                  }
                }
              }
            }
          }
          frame 0, 1, Default {
            # "向下运动"
            n875 = case shown="假" "下降/向右" {
              tunnel: ["下降步伐/um" 0.0 ("X 2")] -> w1602
              tunnel: [0.0 ("X 2") w1647] -> w1601
              tunnel: [0.0 ("Y 2") 0.0 ("Y 2")] -> w1600
              frame False {
              }
              frame True {
                n876 = local read "下降步伐/um"() -> (w1647:dbl)
              }
            }
            n877 = case shown="0" w1593 {
              tunnel: w1594 -> [w1606 _]
              frame 0 {
                n878 = flat-sequence {
                  tunnel: [w1611] -> w1608
                  tunnel: [w1610] -> w1607
                  tunnel: w1606 -> [w1609]
                  tunnel: w1608 -> [w1627]
                  tunnel: w1607 -> [w1626]
                  frame #0 {
                    n879 = VISA Flush I/O Buffer(VISA resource name=w1609) -> (VISA resource name out=w1619:refnum<visa-resource-name>, error out=w1620:errorcluster)  [unwired: 2 in]
                    n880 = Number To Decimal String(number=11 ("数字")) -> (decimal integer string=w1622:string)  [unwired: 1 in]
                    n881 = Concatenate Strings("C," ("字符串"), w1622, "\r") -> (w1624:string)
                    n882 = VISA Write ("VISA写入")(VISA resource name=w1619, write buffer=w1624, error in (no error)=w1620) -> (VISA resource name out=w1613:refnum<visa-resource-name>, error out=w1612:errorcluster)  [unwired: 1 out]
                    n883 = property class="Instr"(reference=w1613, error in=w1612) -> (reference out=w1614:refnum<visa-resource-name>, error out=w1615:errorcluster, "Serial Settings:Number of Bytes at Serial Port"=w1618:u32)
                    n884 = VISA Read(VISA resource name=w1614, byte count=w1618, error in (no error)=w1615) -> (VISA resource name out=w1616:refnum<visa-resource-name>, error out=w1617:errorcluster)  [unwired: 2 out]
                    n885 = VISA Flush I/O Buffer(VISA resource name=w1616, error in (no error)=w1617) -> (VISA resource name out=w1611:refnum<visa-resource-name>, error out=w1610:errorcluster)  [unwired: 1 in]
                  }
                  frame #1 {
                    n886 = disable-structure shown="禁用" {
                      disable-tunnel: w1627 -> [w1629 _]
                      disable-tunnel: w1626 -> [w1628 _]
                      frame Disabled {
                        n887 = Concatenate Strings("D" ("写入缓冲区"), "\r") -> (w1634:string)
                        n888 = VISA Write ("VISA写入")(VISA resource name=w1629, write buffer=w1634, error in (no error)=w1628) -> (VISA resource name out=w1639:refnum<visa-resource-name>, error out=w1637:errorcluster)  [unwired: 1 out]
                        n889 = property class="Instr"(reference=w1639, error in=w1637) -> (reference out=w1636:refnum<visa-resource-name>, error out=w1635:errorcluster, "Serial Settings:Number of Bytes at Serial Port"=w1638:u32)
                        n890 = VISA Read(VISA resource name=w1636, byte count=w1638, error in (no error)=w1635) -> (VISA resource name out=w1633:refnum<visa-resource-name>, error out=w1632:errorcluster)  [unwired: 2 out]
                        n891 = VISA Flush I/O Buffer(VISA resource name=w1633, error in (no error)=w1632) -> ()  [unwired: 1 in, 2 out]
                      }
                      frame Enabled {
                      }
                    }
                  }
                }
              }
              frame 1, Default {
              }
            }
            n892 = call "285_RelMove.vi"("VISA资源名称"=w1604, "Z 2"=w1602, "Y 2"=w1600, "X 2"=w1601) -> ("VISA resource name out 2"=w1605:refnum<visa-resource-name>)  [unwired: 2 in, 5 out]
            n893 = local read "针下降次数"() -> (w1599:i32)
            n894 = Add(x=w1599, y=1) -> (x+y=w1597:i32)
            n895 = Greater?(x=w1597, y=300) -> (0:w1596:bool)
            n896 = case shown="真" w1596 {
              frame False {
              }
              frame True {
                n897 = local write "自动接触"(FALSE ("自动接触")) -> ()
                n898 = One Button Dialog(message="自动接触失败" ("消息")) -> ()  [unwired: 1 in, 1 out]
              }
            }
            n899 = local write "针下降次数"(w1597) -> ()
          }
          frame 11 {
            n900 = local write "自动接触"(FALSE) -> ()
            n901 = local write "自动封接"(TRUE) -> ()
            n902 = local write "自动接触初始"(0) -> ()
            n903 = local write "针下降次数"(0) -> ()
            n904 = One Button Dialog(message="电极已接触细胞" ("消息")) -> ()  [unwired: 1 in, 1 out]
            n905 = Tick Count (ms)() -> (millisecond timer value=→"自动封接开始时间":u32)
          }
        }
      }
    }
    n906 = case shown="真" "升Z轴找针" {
      tunnel: w1064 -> [_ w1122]
      tunnel: w1063 -> [_ w1121]
      frame False {
      }
      frame True {
        # "先上升大步伐，后上升小步伐"
        # "需要计算上升限制\n判断并结束"
        n907 = case shown="2" "升Z轴找针状态机" {
          tunnel: w1122 -> [_ w1144 _]
          tunnel: w1121 -> [w1123 _ _]
          frame 0, Default {
            n908 = flat-sequence {
              tunnel: w1123 -> [w1129]
              frame #0 {
                n909 = local read "物镜下降次数"() -> (w1130:i32)
                n910 = Multiply(x=1 ("数字"), y=w1130) -> (x*y=w1126:i32)
                n911 = Add(x=w1126, y=150) -> (x+y=w1125:i32)
                n912 = call "285_RelMove.vi"("VISA资源名称"=w1129, "Z 2"=w1125, "Y 2"=0.0, "X 2"=0.0) -> ()  [unwired: 2 in, 6 out]
              }
              frame #1 {
                w1133 = u16 1 items=["升Z轴找针初始", "升Z轴找针循环", "升Z轴找针结束"] ("升Z轴找针状态机")
                n913 = local write "升Z轴找针状态机"(w1133) -> ()
                n914 = local write "物镜下降次数"(0) -> ()
                "上升找针次数" <- 0
              }
              frame #2 {
                n915 = case shown="真" "没有细胞" {
                  frame False {
                  }
                  frame True {
                    # "目标坐标"
                    n916 = property on="Image" class="ImageControl"() -> ("ROI"=w1140:T13)  [unwired: 2 in, 2 out]
                    n917 = Unbundle(w1140) -> ("Global Rectangle"=w1138:i32[])  [unwired: 1 out]
                    n918 = Array Subset(array=w1138, index=0 ("索引"), length=2 ("长度")) -> (→"目标坐标":i32[])
                  }
                }
              }
            }
          }
          frame 1 {
            n919 = flat-sequence {
              tunnel: [w1149] -> w1145
              frame #0 {
                n920 = Wait (ms)(milliseconds to wait=u32 100 ("等待时间（毫秒）")) -> ()  [unwired: 1 out]
              }
              frame #1 {
                n921 = local read "没匹配到？"() -> (w1149:bool)
              }
            }
            n922 = case shown="真" w1145 {
              tunnel: w1144 -> [_ w1151]
              frame False {
                w1150 = u16 2 items=["升Z轴找针初始", "升Z轴找针循环", "升Z轴找针结束"] ("升Z轴找针状态机")
                n923 = local write "升Z轴找针状态机"(w1150) -> ()
              }
              frame True {
                n924 = flat-sequence {
                  tunnel: [w1157] -> w1153
                  tunnel: [w1156] -> w1152
                  tunnel: w1151 -> [w1154]
                  tunnel: w1153 -> [w1185]
                  tunnel: w1152 -> [w1184]
                  frame #0 {
                    n925 = VISA Flush I/O Buffer(VISA resource name=w1154) -> (VISA resource name out=w1163:refnum<visa-resource-name>, error out=w1162:errorcluster)  [unwired: 2 in]
                    n926 = Number To Decimal String(number=20 ("数字")) -> (decimal integer string=w1160:string)  [unwired: 1 in]
                    n927 = Concatenate Strings("C," ("字符串"), w1160, "\r") -> (w1158:string)
                    n928 = VISA Write ("VISA写入")(VISA resource name=w1163, write buffer=w1158, error in (no error)=w1162) -> (VISA resource name out=w1169:refnum<visa-resource-name>, error out=w1170:errorcluster)  [unwired: 1 out]
                    n929 = property class="Instr"(reference=w1169, error in=w1170) -> (reference out=w1168:refnum<visa-resource-name>, error out=w1167:errorcluster, "Serial Settings:Number of Bytes at Serial Port"=w1164:u32)
                    n930 = VISA Read(VISA resource name=w1168, byte count=w1164, error in (no error)=w1167) -> (VISA resource name out=w1166:refnum<visa-resource-name>, error out=w1165:errorcluster)  [unwired: 2 out]
                    n931 = VISA Flush I/O Buffer(VISA resource name=w1166, error in (no error)=w1165) -> (VISA resource name out=w1157:refnum<visa-resource-name>, error out=w1156:errorcluster)  [unwired: 1 in]
                  }
                  frame #1 {
                    n932 = local read "上升找针次数"() -> (w1173:i32)
                    n933 = Concatenate Strings("U" ("写入缓冲区"), "\r") -> (w1177:string)
                    n934 = VISA Write ("VISA写入")(VISA resource name=w1185, write buffer=w1177, error in (no error)=w1184) -> (VISA resource name out=w1183:refnum<visa-resource-name>, error out=w1181:errorcluster)  [unwired: 1 out]
                    n935 = Add(x=w1173, y=2) -> (x+y=w1172:i32)
                    n936 = property class="Instr"(reference=w1183, error in=w1181) -> (reference out=w1180:refnum<visa-resource-name>, error out=w1179:errorcluster, "Serial Settings:Number of Bytes at Serial Port"=w1182:u32)
                    n937 = local write "上升找针次数"(w1172) -> ()
                    n938 = VISA Read(VISA resource name=w1180, byte count=w1182, error in (no error)=w1179) -> (VISA resource name out=w1175:refnum<visa-resource-name>, error out=w1174:errorcluster)  [unwired: 2 out]
                    n939 = VISA Flush I/O Buffer(VISA resource name=w1175, error in (no error)=w1174) -> ()  [unwired: 1 in, 2 out]
                  }
                }
              }
            }
            n940 = local read "上升找针次数"() -> (w1143:i32)
            n941 = Greater?(x=w1143, y=500) -> (0:w1141:bool)
            n942 = case shown="真" w1141 {
              frame False {
              }
              frame True {
                n943 = local write "升Z轴找针"(FALSE ("升Z轴找针")) -> ()
                n944 = One Button Dialog(message="没找到针尖" ("消息")) -> ()  [unwired: 1 in, 1 out]
              }
            }
          }
          frame 2 {
            w1186 = u16 0 items=["升Z轴找针初始", "升Z轴找针循环", "升Z轴找针结束"] ("升Z轴找针状态机")
            n945 = local write "升Z轴找针"(FALSE ("升Z轴找针")) -> ()
            n946 = local write "升Z轴找针状态机"(w1186) -> ()
            n947 = local write "针尖移动 2"(TRUE ("针尖自动移动 2")) -> ()
          }
        }
      }
    }
    n948 = local read "没有细胞"() -> (w1059:bool)
    n949 = case shown="真" w1059 {
      frame False {
      }
      frame True {
        # "目标坐标"
        n950 = property on="Image" class="ImageControl"() -> ("ROI"=w1097:T13)  [unwired: 2 in, 2 out]
        n951 = Unbundle(w1097) -> ("Global Rectangle"=w1098:i32[])  [unwired: 1 out]
        n952 = Array Subset(array=w1098, index=0 ("索引"), length=2 ("长度")) -> (w1096:i32[])
        n953 = local write "目标坐标"(w1096) -> ()
      }
    }
    n954 = case shown="真" "保存数据" {
      tunnel: w1087 -> [w1408 w1424]
      tunnel: [w1399 w1424] -> w1075
      tunnel: w1085 -> [w1401 w1423]
      tunnel: w1084 -> [w1397 _]
      tunnel: [w1400 w1423] -> w1076
      tunnel: w1083 -> [w1395 _]
      frame True {
        w1391 = "\t"
        n955 = local read "Resistance(MΩ)"() -> (w1398:dbl)
        n956 = call "285_GetPos.vi"("VISA资源名称"=w1408) -> ("Z"=w1403:dbl, "Y"=w1405:dbl, "X"=w1407:dbl, "VISA资源名称输出"=w1399:refnum<visa-resource-name>)  [unwired: 5 in, 2 out]
        n957 = Quotient & Remainder(x=w1395, y=100) -> (x-y*floor(x/y)=w1393:i32)  [unwired: 1 out]
        n958 = Get Date/Time String(want seconds? (F)=TRUE ("需要秒？(F)")) -> (time string=w1389:string)  [unwired: 2 in, 1 out]
        n959 = Number To Fractional String(number=w1405) -> (F-format string=w1404:string)  [unwired: 3 in]
        n960 = Number To Decimal String(number=w1395) -> (decimal integer string=w1396:string)  [unwired: 1 in]
        n961 = Number To Fractional String(number=w1407) -> (F-format string=w1406:string)  [unwired: 3 in]
        n962 = Number To Fractional String(number=w1403) -> (F-format string=w1402:string)  [unwired: 3 in]
        n963 = Number To Fractional String(number=w1398) -> (F-format string=w1414:string)  [unwired: 3 in]
        n964 = Equal?(x=w1393, y=0) -> (x = y?=w1388:bool)
        n965 = case shown="真" w1388 {
          tunnel: w1397 -> [_ w1418]
          tunnel: w1396 -> [_ w1416]
          frame False {
          }
          frame True {
            n966 = Concatenate Strings("图像" ("字符串"), w1416, ".bmp" ("字符串")) -> (w1420:string)
            n967 = local read "Image"() -> (w1417:T4)
            n968 = Build Path(base path=w1418, name or relative path=w1420) -> (appended path=w1422:path)
            n969 = call-poly "IMAQ Write File 2"("File Path"=w1422, "Image"=w1417) -> ()  [unwired: 8 in, 2 out]
          }
        }
        n970 = Concatenate Strings(w1389, w1391, w1396, w1391, w1391, "X轴：" ("字符串"), w1406, w1391, "Y轴：" ("字符串"), w1404, w1391, "Z轴：" ("字符串"), w1402, w1391, "阻值：" ("字符串"), w1414, "\n") -> (w1409:string)
        n971 = Write to Text File(file (use dialog)=w1401, text=w1409) -> (refnum out=w1400:refnum<file>)  [unwired: 2 in, 2 out]
      }
      frame False {
      }
    }
  }
  n972 = call "IMAQ Dispose"("Image"=w24) -> ()  [unwired: 5 in, 1 out]
  n973 = call "IMAQ Dispose"("Image"=w25) -> ()  [unwired: 5 in, 1 out]
  n974 = call "SetDA.vi"("错误输入（无错误）"=w44, "DevIndex"=w45) -> ("错误输出"=w107:errorcluster, "DevIndex Output"=w108:i32)  [unwired: 8 in]
  n975 = call "SetDA.vi"("错误输入（无错误）"=w107, "DAVolt"=0.0, "DANum"=u8 1, "DevIndex"=w108) -> ("错误输出"=w106:errorcluster, "DevIndex Output"=w105:i32)  [unwired: 6 in]
  n976 = Build Array(w96, w96, w96, w96, w96, w96, w96, w96) -> (w94:bool[])
  n977 = call "SetDA.vi"("错误输入（无错误）"=w106, "DAVolt"=0.0, "DANum"=u8 2, "DevIndex"=w105) -> ("错误输出"=w103:errorcluster, "DevIndex Output"=w104:i32)  [unwired: 6 in]
  n978 = Boolean Array To Number(Boolean array=w94) -> (number=w95:u32)
  n979 = call "SetDA.vi"("错误输入（无错误）"=w103, "DAVolt"=0.0, "DANum"=u8 3, "DevIndex"=w104) -> ("错误输出"=w90:errorcluster, "DevIndex Output"=w91:i32)  [unwired: 6 in]
  n980 = To Unsigned Byte Integer(number=w95) -> (unsigned 8bit integer=w93:u8)
  n981 = call "SetDioOut.vi"("错误输入（无错误）"=w90, "DioOut"=w93, "DioChanSel"=u8 255, "DevIndex"=w91) -> ("错误输出"=w89:errorcluster, "DevIndex Output"=w88:i32)  [unwired: 6 in]
  n982 = call "StopRead.vi"("错误输入（无错误）"=w89, "DevIndex"=w88) -> ("错误输出"=w114:errorcluster, "DevIndex Output"=w115:i32)  [unwired: 8 in]
  n983 = Close File(refnum=w59) -> ()  [unwired: 1 in, 2 out]
  n984 = call "285_Update.vi"("VISA资源名称"=w34) -> ("VISA资源名称 2"=w76:refnum<visa-resource-name>)  [unwired: 9 in, 1 out]
  n985 = VISA Close(VISA resource name=w76) -> ()  [unwired: 1 in, 1 out]
  n986 = call "SetSoftTrig.vi"("错误输入（无错误）"=w114, "Trig"=u8 0, "DevIndex"=w115) -> ("错误输出"=w113:errorcluster, "DevIndex Output"=w111:i32)  [unwired: 7 in]
  n987 = call "ClearTrigger.vi"("错误输入（无错误）"=w113, "DevIndex"=w111) -> ("错误输出"=w112:errorcluster, "DevIndex Output"=w110:i32)  [unwired: 8 in]
  n988 = call "ClearBufs.vi"("错误输入（无错误）"=w112, "DevIndex"=w110) -> ("错误输出"=w116:errorcluster, "DevIndex Output"=w117:i32)  [unwired: 8 in]
  n989 = call "CloseDevice.vi"("错误输入（无错误）"=w116, "DevIndex"=w117) -> ("错误输出"=w74:errorcluster)  [unwired: 8 in, 1 out]
  n990 = Merge Errors(w75, w74) -> (→"错误输出 3":errorcluster)
  n991 = call "285_Update.vi"("VISA资源名称"=w35) -> ("VISA资源名称 2"=w36:refnum<visa-resource-name>)  [unwired: 9 in, 1 out]
  n992 = VISA Close(VISA resource name=w36) -> ()  [unwired: 1 in, 1 out]
